vi "Main UI (ext control).vi"(0 "Serial port":refnum<visa-resource-name>="COM1", 1 "Command":T2, 5 "Data rate (Hz)":dbl=100.0, 7 "Max. num. sensors (override)":u8=64 max=64, 9 "Wait for HW trigger":bool, 11 "Finite samples":bool=TRUE, 12 "N samples":u32=1000, 14 "Error in":errorcluster) -> (4 "P data (mode 0)":T8[](array[typedef]), 15 "Error out":errorcluster)   [LabVIEW 2020]
doc: "User interface for 64 pressure multiplexer system designed by Paul Nathan, 02/2016"
uses:
  Ctls/System status.ctl
  Ctls/Environmental state values.ctl
  Ctls/Inertial state values.ctl
  Ctls/AccelGyro constants.ctl
  Ctls/Pressure sensor constants.ctl
  Ctls/Cmd list.ctl
  Ctls/Data values, Mode 0 (for datalog).ctl
  Ctls/All state values (for datalog).ctl
  Ctls/Cmd str.ctl
  Ctls/Data values, Mode 1 (for datalog).ctl
panel:
  in  "Main tabs":T1(tab)
  in  "Env. period (ms)":i32=1000 min=0
  out "ACK 8":bool caption="ACK"
  out "ACK 7":bool caption="ACK"
  out "ACK 6":bool caption="ACK"
  out "AccelGyro constants":T3={"gyrRange"=125.0, "accRange"=2.0, "gx offset"=0.0, "gy offset"=0.0, "gz offset"=0.0, "ax offset"=0.0, "ay offset"=0.0, "az offset"=0.0, "axyz scale"=1.0} {"axyz scale" format="%#_4f"; "az offset" format="%#_4f"; "ay offset" format="%#_4f"; "ax offset" format="%#_4f"; "gz offset" format="%#_4f"; "gy offset" format="%#_4f"; "gx offset" format="%#_4f"; "gyrRange" format="%#_4f"; "accRange" format="%#_4f"}
  out "Faulty sensors":i32[](array[numeric])
  out "ACK 5":bool caption="ACK"
  out "Active sensors":i32[](array[numeric])
  out "ACK 4":bool caption="ACK"
  in  "Gyro. rate (Hz)":u8(ring) items=["6.25", "12.5", "25", "50", "100", "200", "400", "800", "1600", "3200"]
  in  "Gyro. range (dps)":u8(ring) items=["+/- 125", "+/- 250", "+/- 500", "+/- 1000", "+/- 2000"]
  in  "Accel. rate (Hz)":u8(ring)=1 items=["3.125", "6.25", "12.5", "25", "50", "100", "200", "400", "800", "1600"]
  in  "Accel. range (g)":u8(ring) items=["+/- 2", "+/- 4", "+/- 8", "+/- 16"]
  out "Inertial state values":T4 {"w_z (dps)" format="%#_4f"; "a_y (g)" format="%#_4f"; "a_z (g)" format="%#_4f"; "w_y (dps)" format="%#_4f"; "a_x (g)" format="%#_4f"; "Sensor temp. (degC)" format="%#.2f"; "w_x (dps)" format="%#_4f"}
  out "Environmental state values":T5 {"Dew point (degC)" format="%#.2f"; "Density (kg/m^3)" format="%#.3f"; "Pressure alt. (m)" format="%#.2f"; "Density alt. (m)" format="%#.2f"; "Rel. Humidity (%)" format="%#.2f"; "P_atmos (Pa)" format="%#_6f"; "Sensor temp. (degC)" format="%#.2f"; "Thermistor (degC)" format="%#.2f"}
  out "System status":T6
  out "ACK 3":bool caption="ACK"
  out "ACK 1":bool caption="ACK"
  in  "Data mode":u8(ring) items=["P", "P & T"]
  out "ACK 2":bool caption="ACK"
  out "Main Power":bool
  out "L_data (bytes)":u16
  out "Serial no.":u16 format="%04x"
  out "Active pressure sensor constants":T7[](array[typedef])
  out "Streaming":bool
  out "Clock drift":bool
  out "Sensor temperatures time trace (Mode \"P & T\" only)":sgl[][](graph)
  out "Pressures time trace":sgl[][](graph)
  in  "Stop streaming":bool
  out "Stale samples flag":u8[][](graph)
  out "Samples acquired":u32
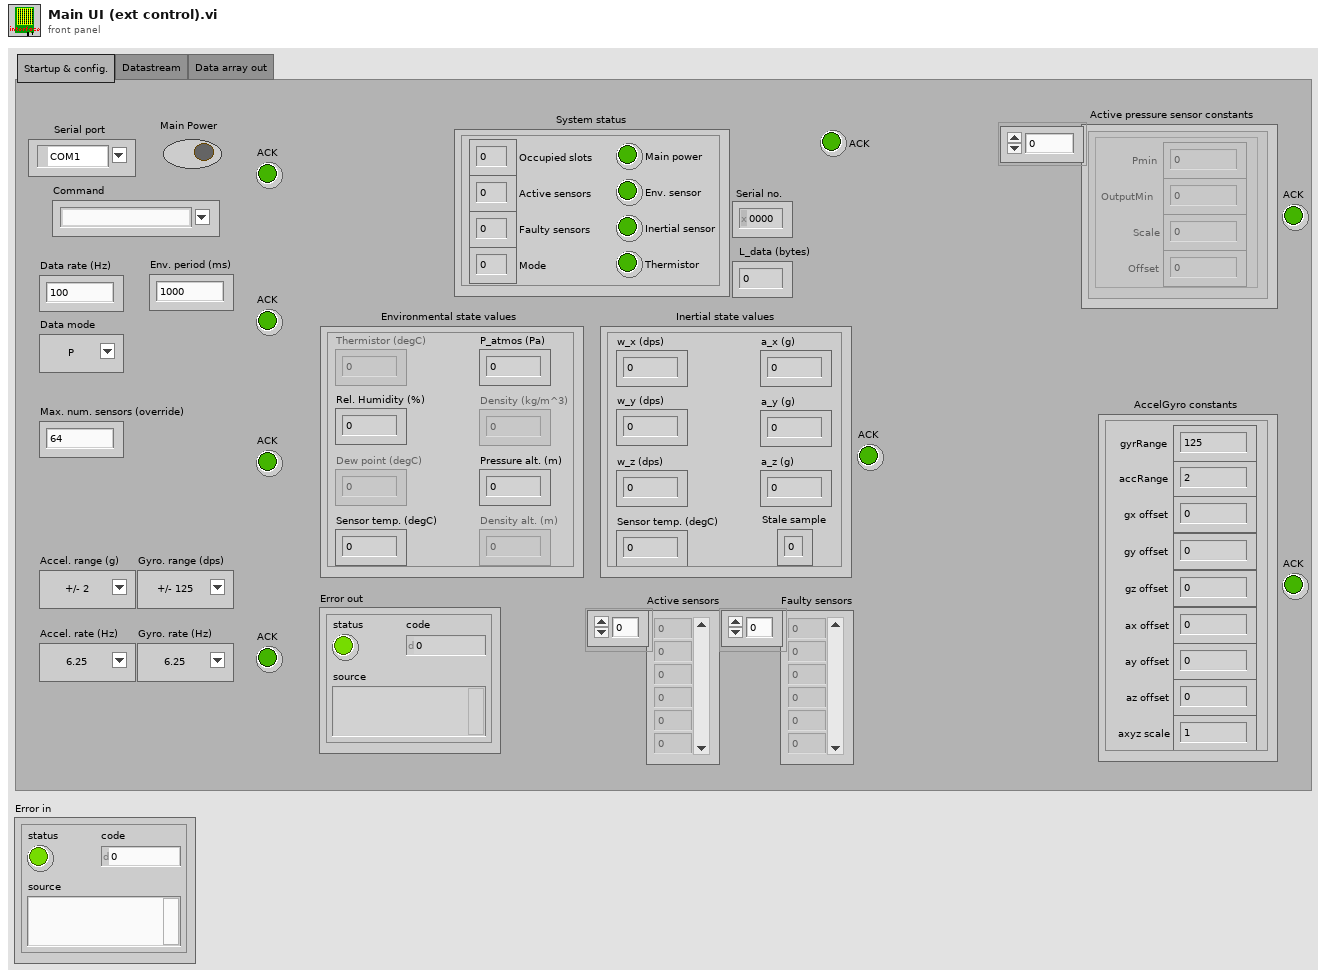
[diagram p1: front panel]
types:
  T1 = enum32{"Startup & config.", "Datastream", "Data array out"}
  T2 = typedef "Cmd list.ctl" = string
  T3 = typedef "AccelGyro constants.ctl" = cluster{"gyrRange":sgl, "accRange":sgl, "gx offset":sgl, "gy offset":sgl, "gz offset":sgl, "ax offset":sgl, "ay offset":sgl, "az offset":sgl, "axyz scale":sgl}
  T4 = typedef "Inertial state values.ctl" = cluster{"w_x (dps)":sgl, "w_y (dps)":sgl, "w_z (dps)":sgl, "a_x (g)":sgl, "a_y (g)":sgl, "a_z (g)":sgl, "Stale sample":u8, "Sensor temp. (degC)":sgl}
  T5 = typedef "Environmental state values.ctl" = cluster{"Thermistor (degC)":sgl, "Sensor temp. (degC)":sgl, "P_atmos (Pa)":sgl, "Rel. Humidity (%)":sgl, "Density (kg/m^3)":sgl, "Dew point (degC)":sgl, "Pressure alt. (m)":sgl, "Density alt. (m)":sgl}
  T6 = typedef "System status.ctl" = cluster{"Main power":bool, "Occupied slots":u8, "Active sensors":u8, "Faulty sensors":u8, "Env. sensor":bool, "Inertial sensor":bool, "Thermistor":bool, "Mode":u8}
  T7 = typedef "Pressure sensor constants.ctl" = cluster{"Pmin":sgl, "OutputMin":sgl, "Scale":sgl, "Offset":sgl}
  T8 = typedef "Data values, Mode 0 (for datalog).ctl" = cluster{"Time Stamp":timestamp, "dt (us)":sgl, "dt_warn":u8, "Pressures":sgl[], "Statuses":u8[]}
  T9 = typedef "All state values (for datalog).ctl" = cluster{"Time Stamp":timestamp, "dt (ms)":i32, "Environmental state values":T5, "Inertial state values":T4}
  T10 = typedef "Cmd str.ctl" = string
  T11 = typedef "Data values, Mode 1 (for datalog).ctl" = cluster{"Time Stamp":timestamp, "dt (us)":sgl, "dt_warn":u8, "Pressures":sgl[], "Die temps.":sgl[], "Statuses":u8[]}
  T12 = enum8{"Enabled", "Disabled", "Disabled and Grayed Out"}
  T13 = typedef "EEPROM page.ctl" = cluster{"Pmin (Pa)":sgl, "Pmax (Pa)":sgl, "maxCount":u16, "minCount":u16, "Poffset (Pa)":sgl}
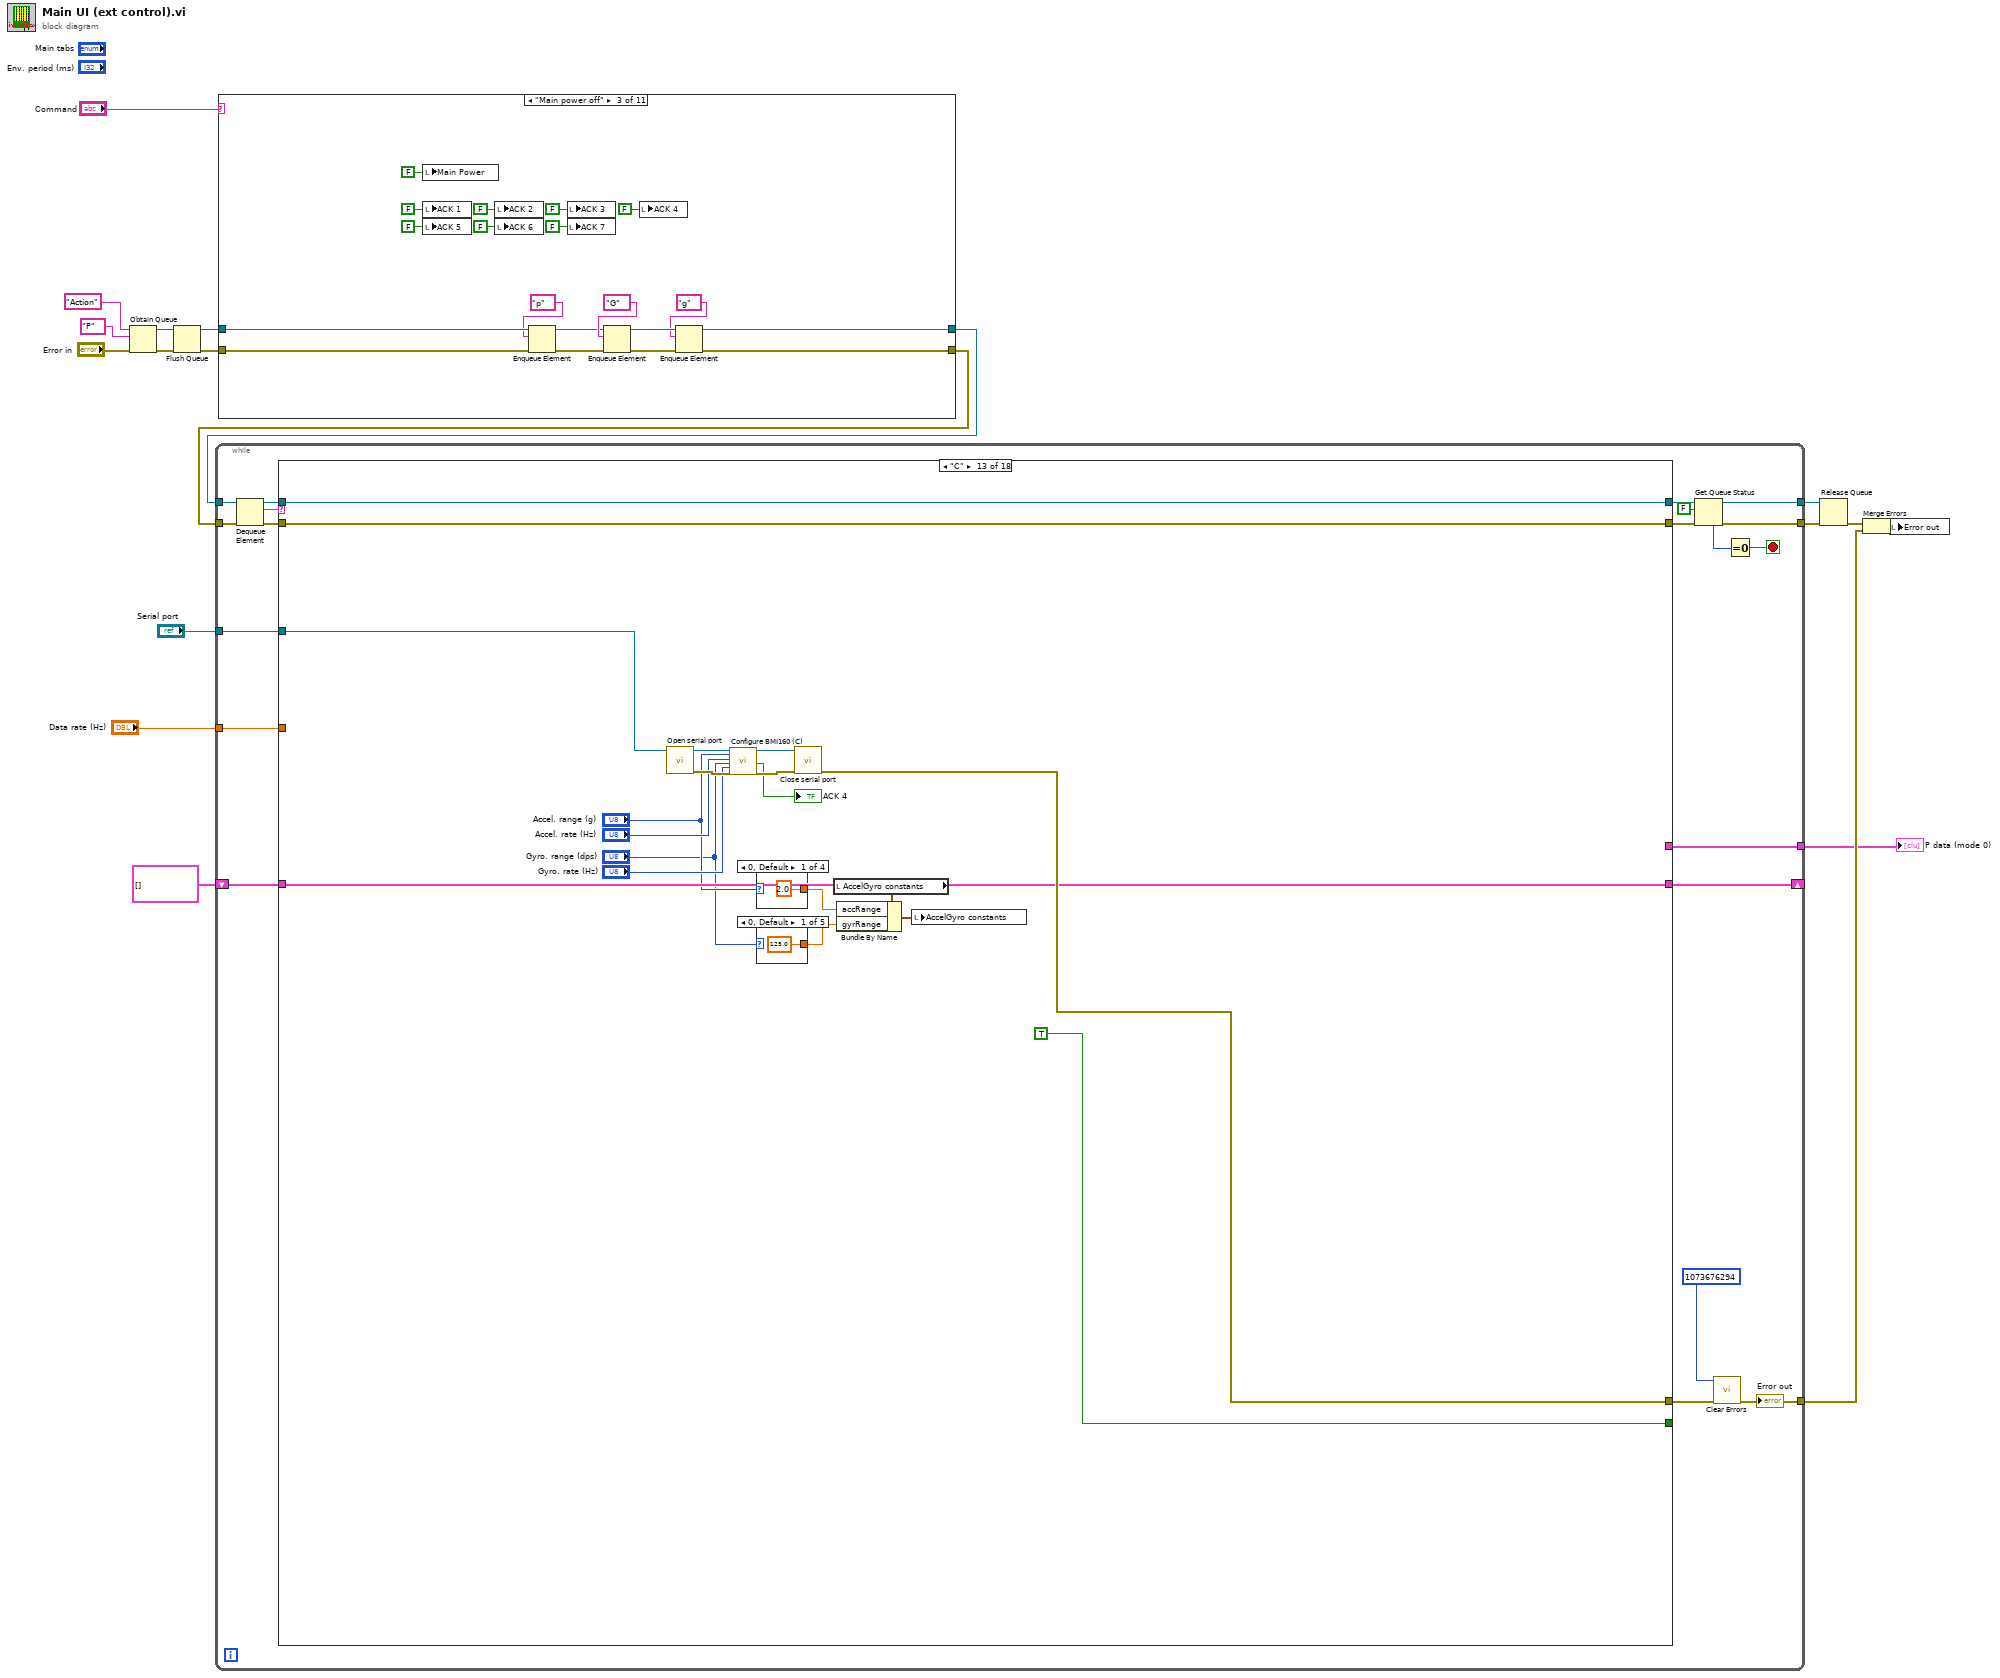
[diagram p0: block diagram]
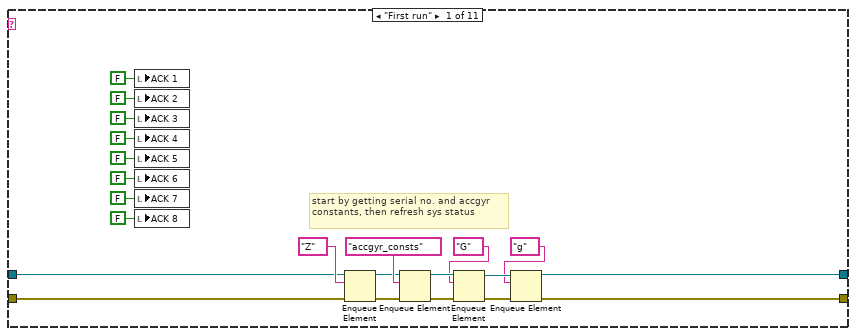
[diagram p2: hidden frame]
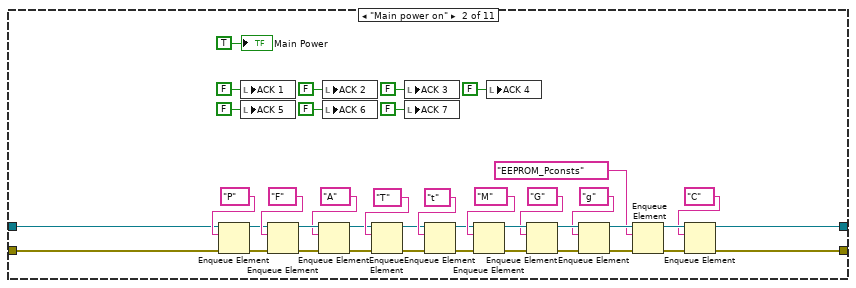
[diagram p3: hidden frame]
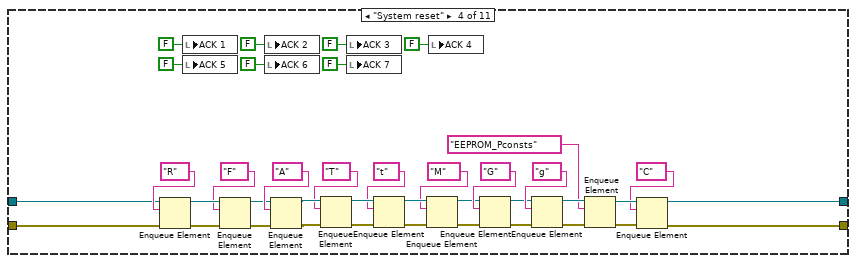
[diagram p4: hidden frame]
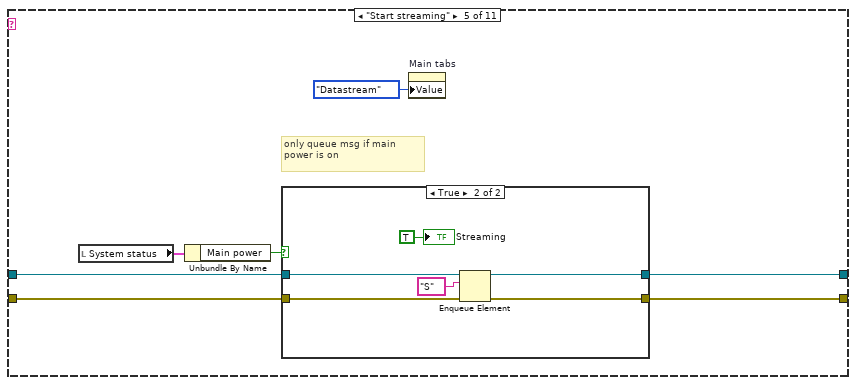
[diagram p5: hidden frame]
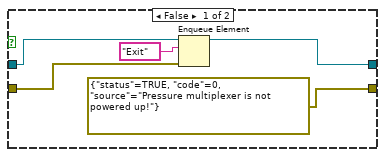
[diagram p6: hidden frame]
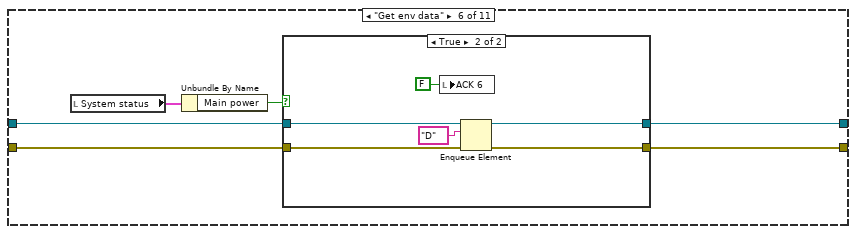
[diagram p7: hidden frame]
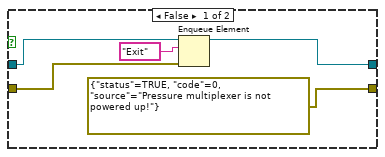
[diagram p8: hidden frame]
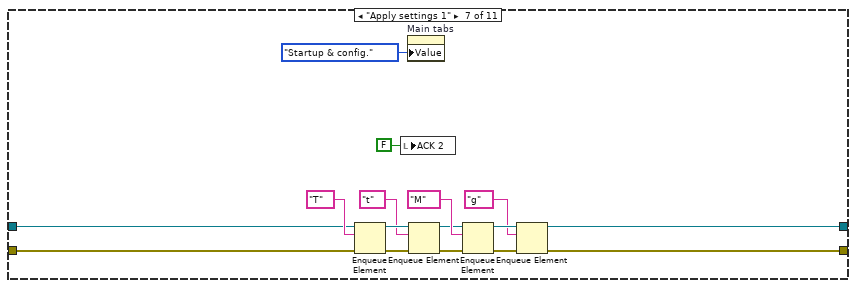
[diagram p9: hidden frame]
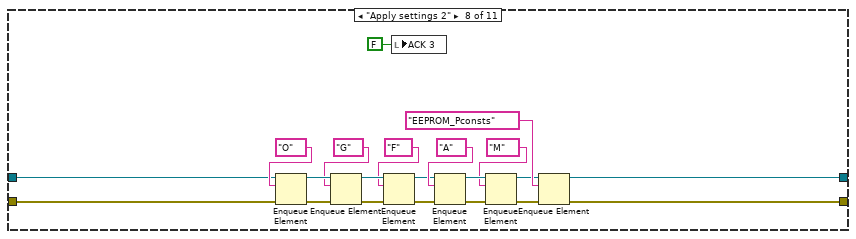
[diagram p10: hidden frame]
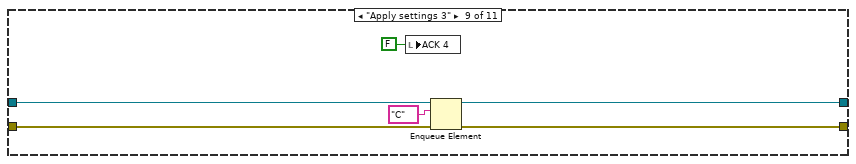
[diagram p11: hidden frame]
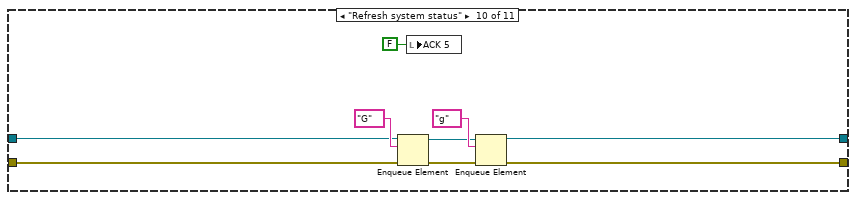
[diagram p12: hidden frame]
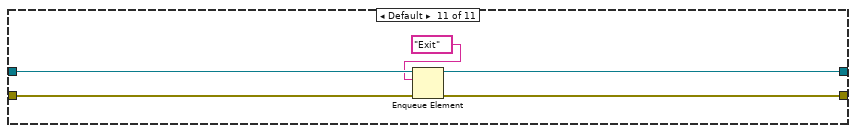
[diagram p13: hidden frame]
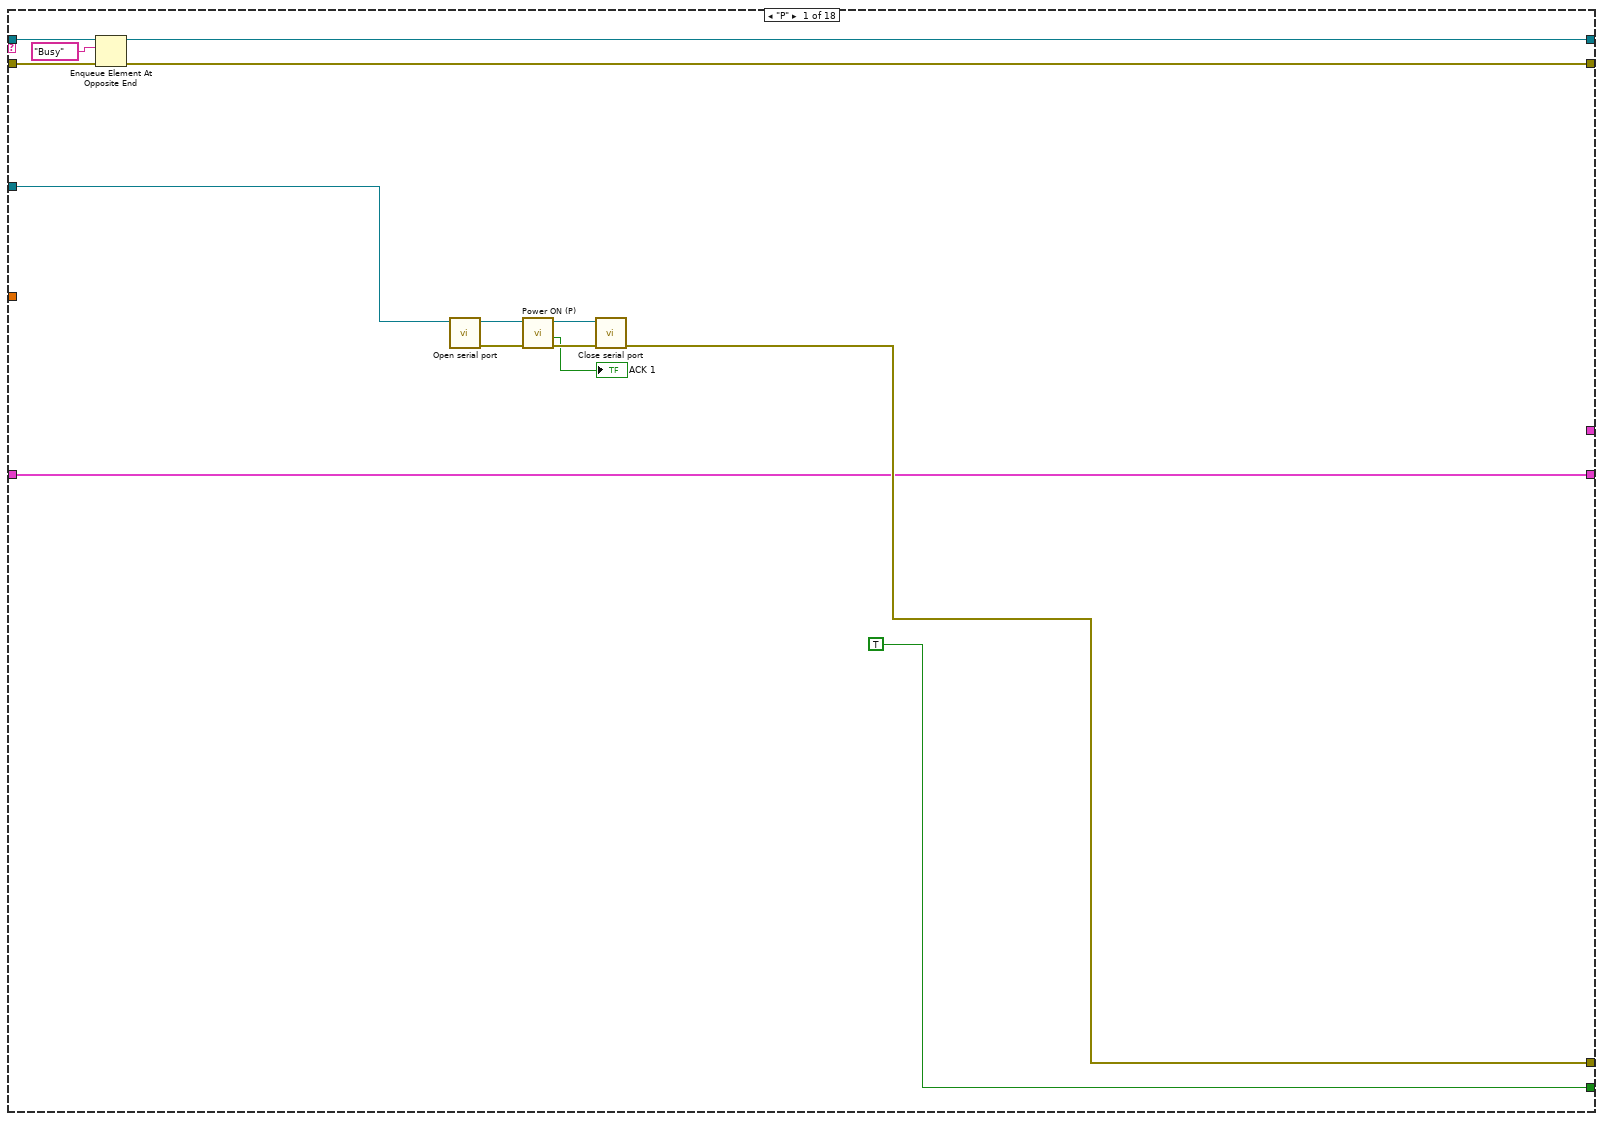
[diagram p14: hidden frame]
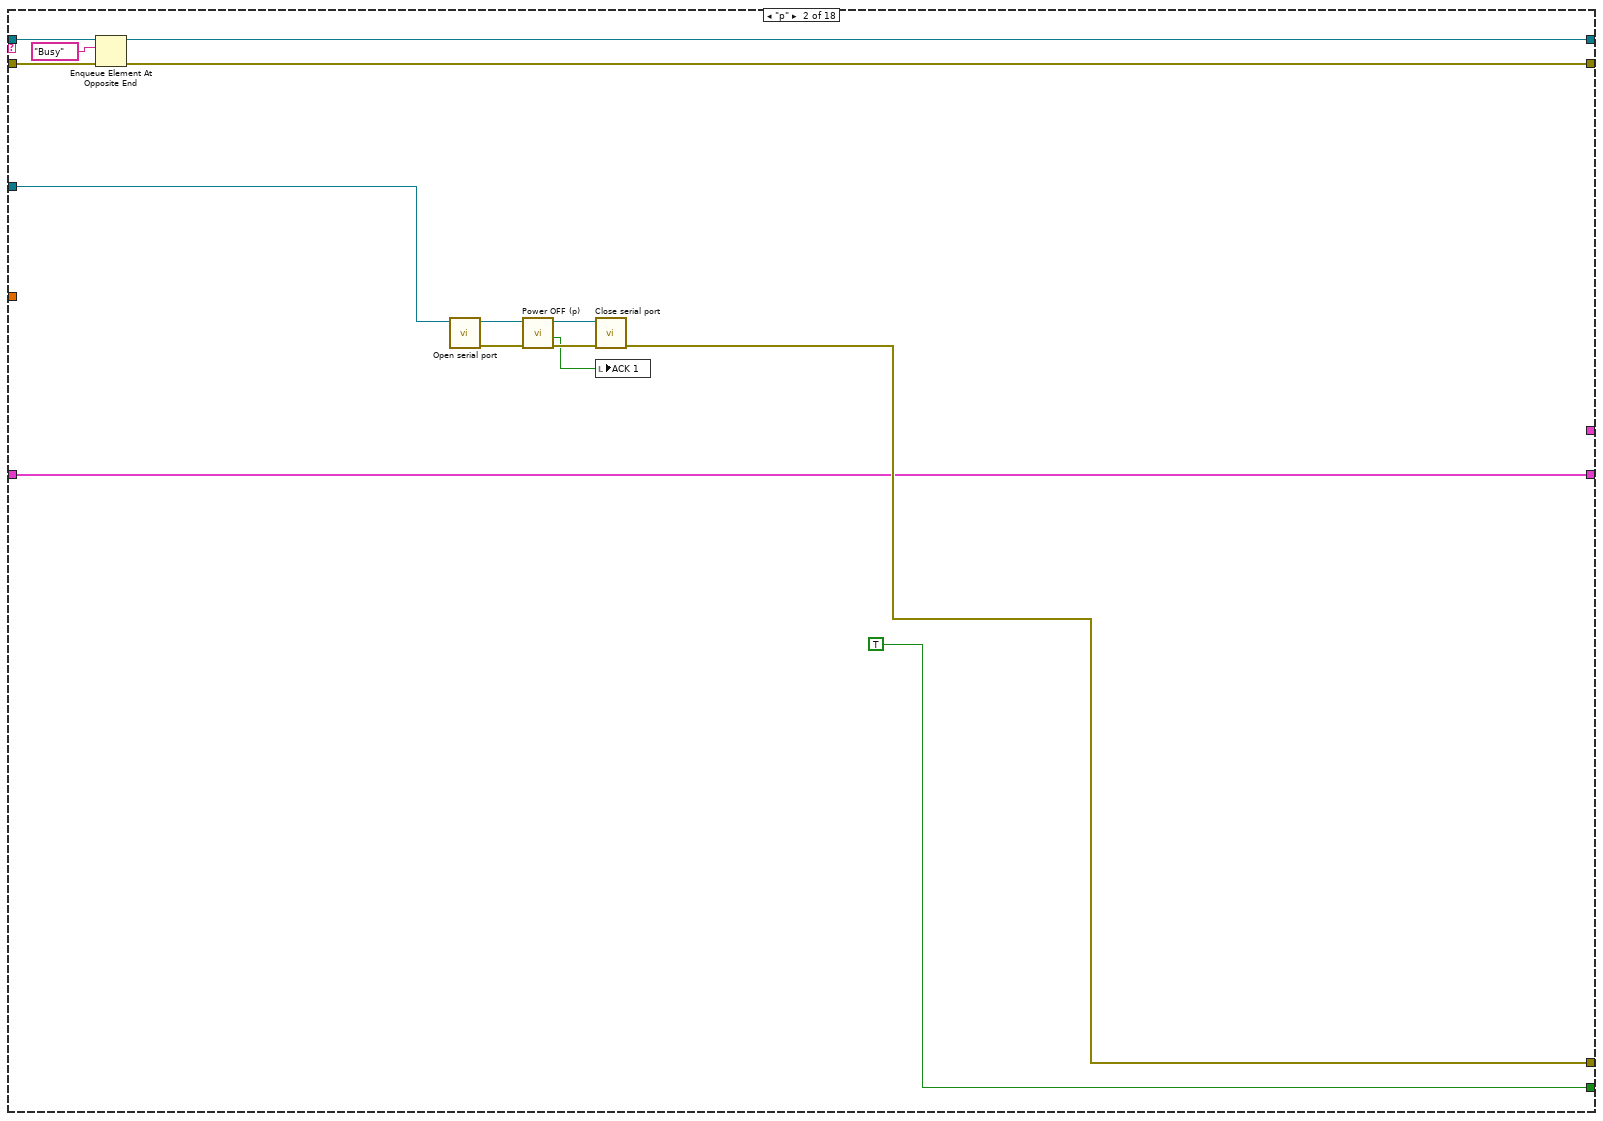
[diagram p15: hidden frame]
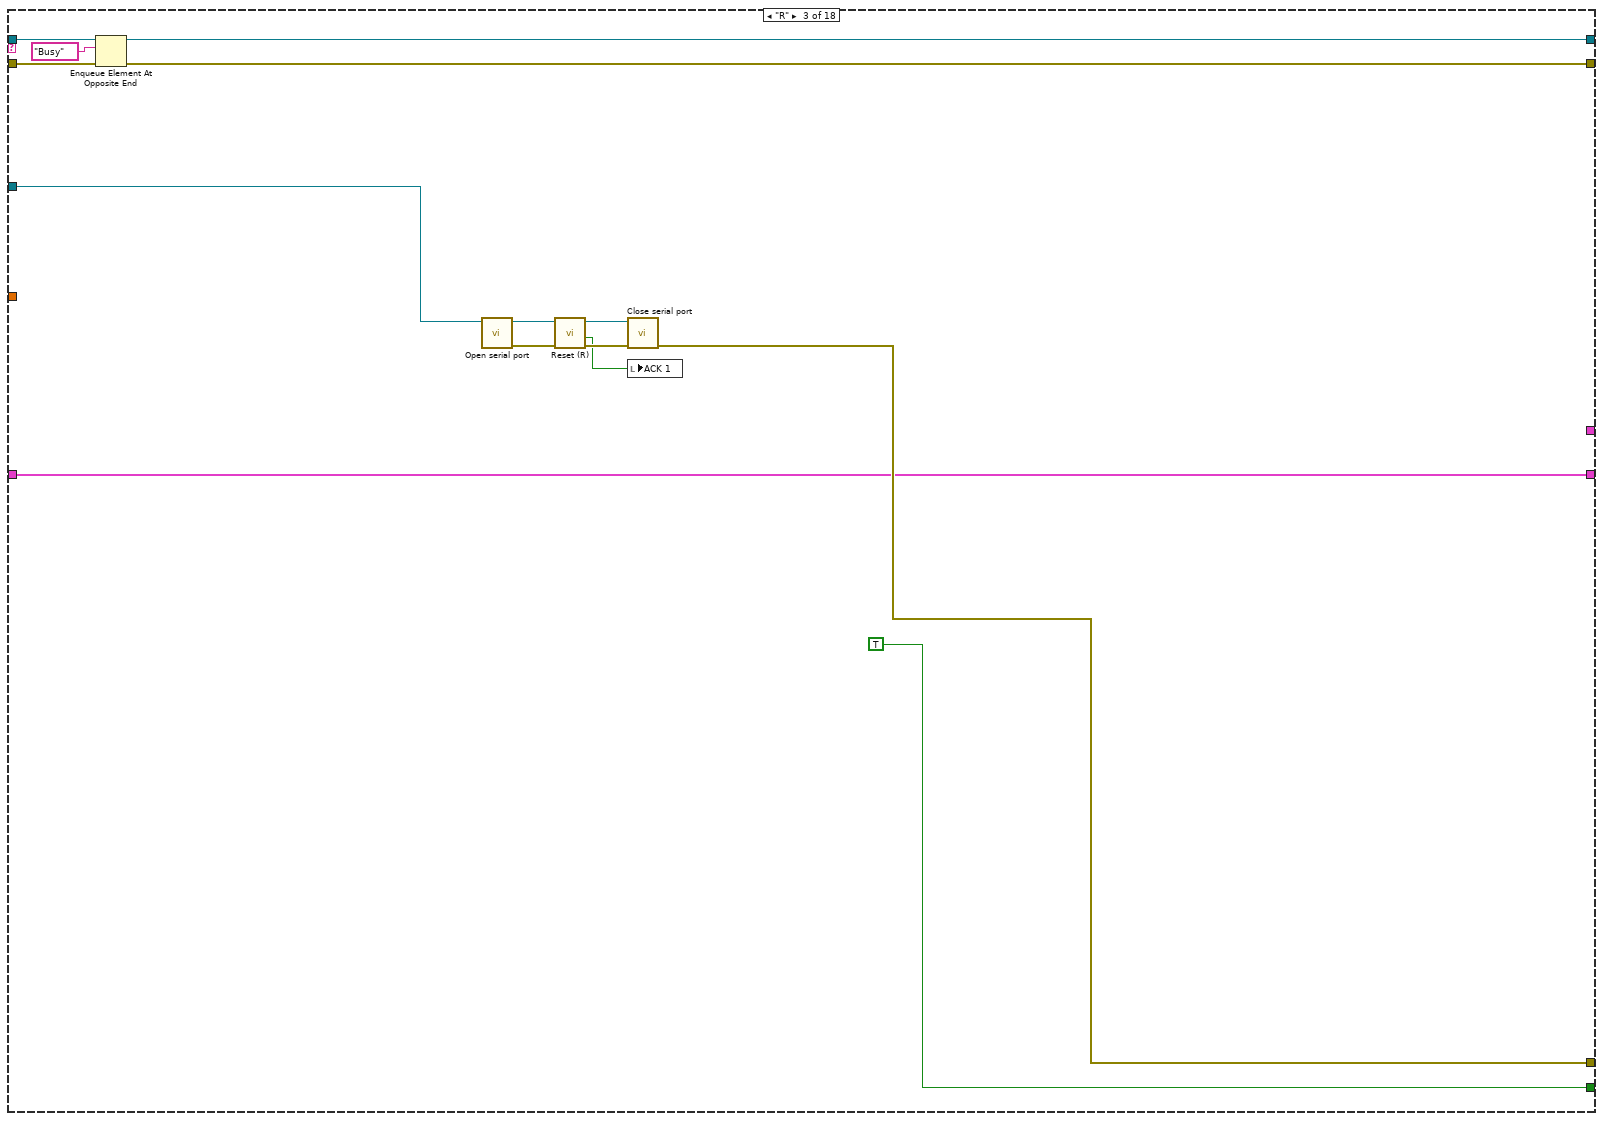
[diagram p16: hidden frame]
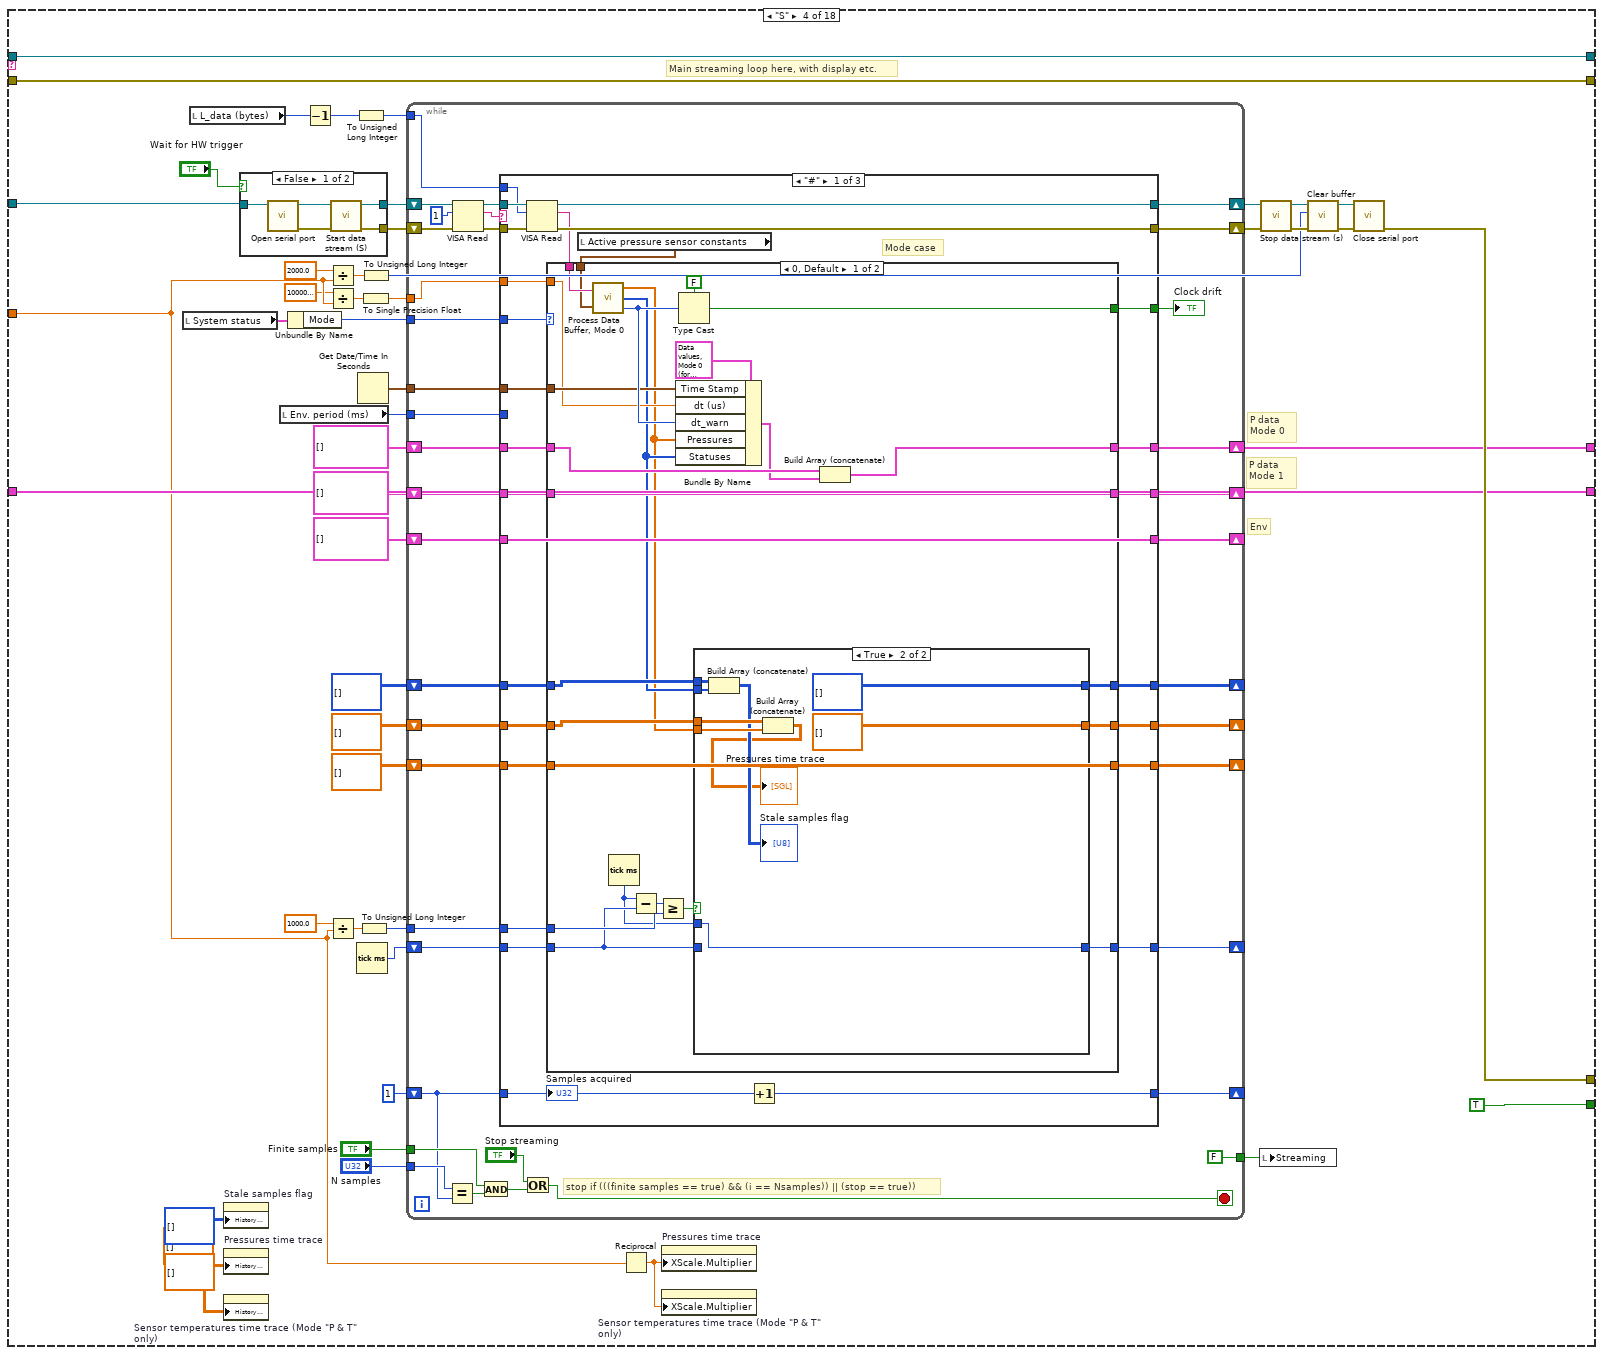
[diagram p17: hidden frame]
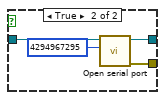
[diagram p18: hidden frame]
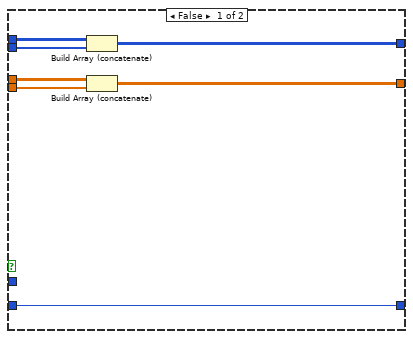
[diagram p19: hidden frame]
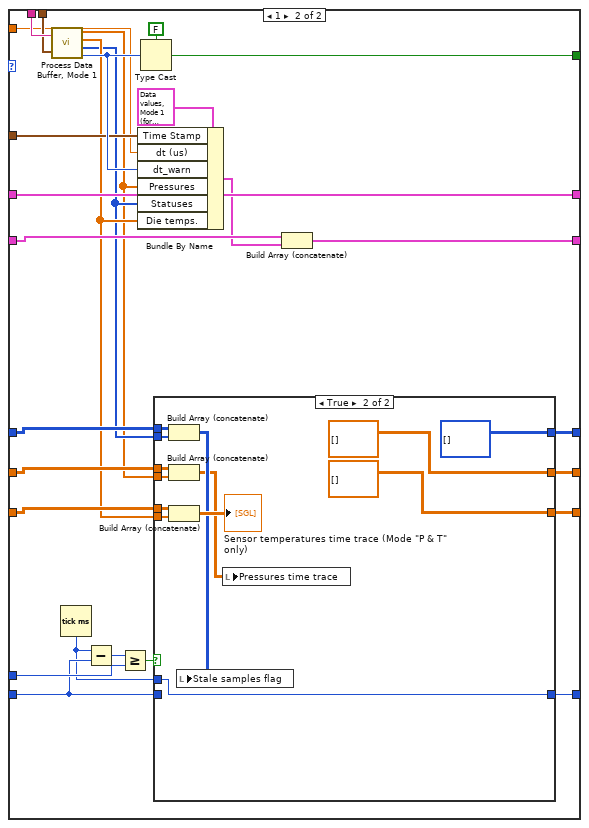
[diagram p20: hidden frame]
diagram:
  n1 = Obtain Queue(name (unnamed)="Action", element data type=T10 "P" ("Cmd"), error in (no error)="Error in") -> (queue out=w18:refnum<queue>, error out=w17:errorcluster)  [unwired: 2 in, 1 out]
  n2 = Flush Queue(queue=w18, error in (no error)=w17) -> (queue out=w6:refnum<queue>, error out=w5:errorcluster)  [unwired: 1 out]
  n3 = case shown="\"Main power off\"" "Command" {
    tunnel: [w29 w52 w92 w109 w141 w160 w178 w193 w214 w219 w227] -> w9
    tunnel: w5 -> [w30 w79 w99 w110 w144 w161 w179 w194 w215 w222 w231]
    tunnel: w6 -> [w31 w80 w100 w111 w143 w162 w180 w195 w216 w221 w230]
    tunnel: [w28 w51 w91 w108 w142 w159 w177 w192 w213 w220 w228] -> w8
    frame "First run" {
      # "start by getting serial no. and accgyr constants, then refresh sys status"
      n4 = local write "ACK 1"(FALSE ("ACK 8")) -> ()
      n5 = local write "ACK 2"(FALSE ("ACK 6")) -> ()
      n6 = local write "ACK 3"(FALSE ("ACK 8")) -> ()
      n7 = local write "ACK 4"(FALSE ("Done")) -> ()
      n8 = local write "ACK 5"(FALSE ("ACK 8")) -> ()
      n9 = local write "ACK 6"(FALSE ("ACK 6")) -> ()
      n10 = local write "ACK 7"(FALSE ("ACK 6")) -> ()
      n11 = local write "ACK 8"(FALSE ("ACK 8")) -> ()
      n12 = Enqueue Element(queue=w31, element=T10 "Z", error in (no error)=w30) -> (queue out=w33:refnum<queue>, error out=w34:errorcluster)  [unwired: 1 in, 1 out]
      n13 = Enqueue Element(queue=w33, element=T10 "accgyr_consts", error in (no error)=w34) -> (queue out=w40:refnum<queue>, error out=w41:errorcluster)  [unwired: 1 in, 1 out]
      n14 = Enqueue Element(queue=w40, element=T10 "G" ("Cmd"), error in (no error)=w41) -> (queue out=w38:refnum<queue>, error out=w37:errorcluster)  [unwired: 1 in, 1 out]
      n15 = Enqueue Element(queue=w38, element=T10 "g" ("Cmd"), error in (no error)=w37) -> (queue out=w28:refnum<queue>, error out=w29:errorcluster)  [unwired: 1 in, 1 out]
    }
    frame "Main power on" {
      n16 = Enqueue Element(queue=w80, element=T10 "P" ("Cmd"), error in (no error)=w79) -> (queue out=w73:refnum<queue>, error out=w72:errorcluster)  [unwired: 1 in, 1 out]
      n17 = local write "ACK 1"(FALSE ("ACK 1")) -> ()
      n18 = local write "ACK 5"(FALSE ("ACK 8")) -> ()
      n19 = Enqueue Element(queue=w73, element=T10 "F" ("Cmd"), error in (no error)=w72) -> (queue out=w77:refnum<queue>, error out=w78:errorcluster)  [unwired: 1 in, 1 out]
      n20 = Enqueue Element(queue=w77, element=T10 "A" ("Cmd"), error in (no error)=w78) -> (queue out=w58:refnum<queue>, error out=w57:errorcluster)  [unwired: 1 in, 1 out]
      n21 = local write "ACK 2"(FALSE ("ACK 6")) -> ()
      n22 = local write "ACK 6"(FALSE ("ACK 6")) -> ()
      n23 = Enqueue Element(queue=w58, element=T10 "T" ("Cmd"), error in (no error)=w57) -> (queue out=w60:refnum<queue>, error out=w59:errorcluster)  [unwired: 1 in, 1 out]
      n24 = local write "ACK 3"(FALSE ("ACK 8")) -> ()
      n25 = local write "ACK 7"(FALSE ("ACK 6")) -> ()
      n26 = Enqueue Element(queue=w60, element=T10 "t" ("Cmd"), error in (no error)=w59) -> (queue out=w55:refnum<queue>, error out=w56:errorcluster)  [unwired: 1 in, 1 out]
      n27 = Enqueue Element(queue=w55, element=T10 "M" ("Cmd"), error in (no error)=w56) -> (queue out=w69:refnum<queue>, error out=w68:errorcluster)  [unwired: 1 in, 1 out]
      n28 = local write "ACK 4"(FALSE ("Done")) -> ()
      n29 = Enqueue Element(queue=w69, element=T10 "G" ("Cmd"), error in (no error)=w68) -> (queue out=w70:refnum<queue>, error out=w71:errorcluster)  [unwired: 1 in, 1 out]
      n30 = Enqueue Element(queue=w70, element=T10 "g" ("Cmd"), error in (no error)=w71) -> (queue out=w65:refnum<queue>, error out=w64:errorcluster)  [unwired: 1 in, 1 out]
      n31 = Enqueue Element(queue=w65, element=T10 "EEPROM_Pconsts" ("Cmd"), error in (no error)=w64) -> (queue out=w54:refnum<queue>, error out=w53:errorcluster)  [unwired: 1 in, 1 out]
      n32 = Enqueue Element(queue=w54, element=T10 "C" ("Cmd"), error in (no error)=w53) -> (queue out=w51:refnum<queue>, error out=w52:errorcluster)  [unwired: 1 in, 1 out]
      "Main Power" <- TRUE ("Main Power")
    }
    frame "Main power off" {
      n33 = local write "Main Power"(FALSE ("Main Power")) -> ()
      n34 = local write "ACK 1"(FALSE ("ACK 1")) -> ()
      n35 = local write "ACK 5"(FALSE ("ACK 8")) -> ()
      n36 = local write "ACK 2"(FALSE ("ACK 6")) -> ()
      n37 = local write "ACK 6"(FALSE ("ACK 6")) -> ()
      n38 = Enqueue Element(queue=w100, element=T10 "p" ("Cmd"), error in (no error)=w99) -> (queue out=w96:refnum<queue>, error out=w95:errorcluster)  [unwired: 1 in, 1 out]
      n39 = local write "ACK 3"(FALSE ("ACK 8")) -> ()
      n40 = local write "ACK 7"(FALSE ("ACK 6")) -> ()
      n41 = Enqueue Element(queue=w96, element=T10 "G" ("Cmd"), error in (no error)=w95) -> (queue out=w94:refnum<queue>, error out=w93:errorcluster)  [unwired: 1 in, 1 out]
      n42 = local write "ACK 4"(FALSE ("Done")) -> ()
      n43 = Enqueue Element(queue=w94, element=T10 "g" ("Cmd"), error in (no error)=w93) -> (queue out=w91:refnum<queue>, error out=w92:errorcluster)  [unwired: 1 in, 1 out]
    }
    frame "System reset" {
      n44 = Enqueue Element(queue=w111, element=T10 "R" ("Cmd"), error in (no error)=w110) -> (queue out=w123:refnum<queue>, error out=w124:errorcluster)  [unwired: 1 in, 1 out]
      n45 = local write "ACK 1"(FALSE ("ACK 1")) -> ()
      n46 = local write "ACK 5"(FALSE ("ACK 8")) -> ()
      n47 = Enqueue Element(queue=w123, element=T10 "F" ("Cmd"), error in (no error)=w124) -> (queue out=w115:refnum<queue>, error out=w125:errorcluster)  [unwired: 1 in, 1 out]
      n48 = local write "ACK 2"(FALSE ("ACK 6")) -> ()
      n49 = local write "ACK 6"(FALSE ("ACK 6")) -> ()
      n50 = Enqueue Element(queue=w115, element=T10 "A" ("Cmd"), error in (no error)=w125) -> (queue out=w133:refnum<queue>, error out=w134:errorcluster)  [unwired: 1 in, 1 out]
      n51 = Enqueue Element(queue=w133, element=T10 "T" ("Cmd"), error in (no error)=w134) -> (queue out=w131:refnum<queue>, error out=w132:errorcluster)  [unwired: 1 in, 1 out]
      n52 = local write "ACK 3"(FALSE ("ACK 8")) -> ()
      n53 = local write "ACK 7"(FALSE ("ACK 6")) -> ()
      n54 = Enqueue Element(queue=w131, element=T10 "t" ("Cmd"), error in (no error)=w132) -> (queue out=w135:refnum<queue>, error out=w136:errorcluster)  [unwired: 1 in, 1 out]
      n55 = Enqueue Element(queue=w135, element=T10 "M" ("Cmd"), error in (no error)=w136) -> (queue out=w119:refnum<queue>, error out=w126:errorcluster)  [unwired: 1 in, 1 out]
      n56 = local write "ACK 4"(FALSE ("Done")) -> ()
      n57 = Enqueue Element(queue=w119, element=T10 "G" ("Cmd"), error in (no error)=w126) -> (queue out=w118:refnum<queue>, error out=w127:errorcluster)  [unwired: 1 in, 1 out]
      n58 = Enqueue Element(queue=w118, element=T10 "g" ("Cmd"), error in (no error)=w127) -> (queue out=w122:refnum<queue>, error out=w128:errorcluster)  [unwired: 1 in, 1 out]
      n59 = Enqueue Element(queue=w122, element=T10 "EEPROM_Pconsts" ("Cmd"), error in (no error)=w128) -> (queue out=w138:refnum<queue>, error out=w139:errorcluster)  [unwired: 1 in, 1 out]
      n60 = Enqueue Element(queue=w138, element=T10 "C" ("Cmd"), error in (no error)=w139) -> (queue out=w108:refnum<queue>, error out=w109:errorcluster)  [unwired: 1 in, 1 out]
    }
    frame "Start streaming" {
      # "only queue msg if main power is on"
      n61 = local read "System status"() -> (w146:T6)
      n62 = Unbundle By Name(w146) -> ("Main power"=w145:bool)
      n63 = case shown="True" w145 {
        tunnel: w143 -> [w149 w156]
        tunnel: w144 -> [w147 w155]
        tunnel: [w148 w153] -> w142
        tunnel: [errorcluster {"status"=TRUE, "code"=0, "source"="Pressure multiplexer is not powered up!"} ("error out") w154] -> w141
        frame False {
          n64 = Enqueue Element(queue=w149, element=T10 "Exit" ("Cmd"), error in (no error)=w147) -> (queue out=w148:refnum<queue>)  [unwired: 1 in, 2 out]
        }
        frame True {
          n65 = Enqueue Element(queue=w156, element=T10 "S" ("Cmd"), error in (no error)=w155) -> (queue out=w153:refnum<queue>, error out=w154:errorcluster)  [unwired: 1 in, 1 out]
          "Streaming" <- TRUE ("Streaming")
        }
      }
      n66 = property on="Main tabs" class="TabCtl (strict)"("Value"=T1."Datastream" ("Main tabs")) -> ()  [unwired: 2 in, 2 out]
    }
    frame "Get env data" {
      n67 = local read "System status"() -> (w163:T6)
      n68 = Unbundle By Name(w163) -> ("Main power"=w158:bool)
      n69 = case shown="True" w158 {
        tunnel: w162 -> [w166 w173]
        tunnel: w161 -> [w164 w172]
        tunnel: [w165 w170] -> w159
        tunnel: [errorcluster {"status"=TRUE, "code"=0, "source"="Pressure multiplexer is not powered up!"} ("error out") w171] -> w160
        frame False {
          n70 = Enqueue Element(queue=w166, element=T10 "Exit" ("Cmd"), error in (no error)=w164) -> (queue out=w165:refnum<queue>)  [unwired: 1 in, 2 out]
        }
        frame True {
          n71 = local write "ACK 6"(FALSE ("ACK 6")) -> ()
          n72 = Enqueue Element(queue=w173, element=T10 "D" ("Cmd"), error in (no error)=w172) -> (queue out=w170:refnum<queue>, error out=w171:errorcluster)  [unwired: 1 in, 1 out]
        }
      }
    }
    frame "Apply settings 1" {
      n73 = Enqueue Element(queue=w180, element=T10 "T" ("Cmd"), error in (no error)=w179) -> (queue out=w183:refnum<queue>, error out=w184:errorcluster)  [unwired: 1 in, 1 out]
      n74 = local write "ACK 2"(FALSE ("ACK 6")) -> ()
      n75 = property on="Main tabs" class="TabCtl (strict)"("Value"=T1."Startup & config." ("Main tabs")) -> ()  [unwired: 2 in, 2 out]
      n76 = Enqueue Element(queue=w183, element=T10 "t" ("Cmd"), error in (no error)=w184) -> (queue out=w186:refnum<queue>, error out=w185:errorcluster)  [unwired: 1 in, 1 out]
      n77 = Enqueue Element(queue=w186, element=T10 "M" ("Cmd"), error in (no error)=w185) -> (queue out=w189:refnum<queue>, error out=w190:errorcluster)  [unwired: 1 in, 1 out]
      n78 = Enqueue Element(queue=w189, element=T10 "g" ("Cmd"), error in (no error)=w190) -> (queue out=w177:refnum<queue>, error out=w178:errorcluster)  [unwired: 1 in, 1 out]
    }
    frame "Apply settings 2" {
      n79 = Enqueue Element(queue=w195, element=T10 "O" ("Cmd"), error in (no error)=w194) -> (queue out=w198:refnum<queue>, error out=w199:errorcluster)  [unwired: 1 in, 1 out]
      n80 = Enqueue Element(queue=w198, element=T10 "G" ("Cmd"), error in (no error)=w199) -> (queue out=w210:refnum<queue>, error out=w211:errorcluster)  [unwired: 1 in, 1 out]
      n81 = Enqueue Element(queue=w210, element=T10 "F" ("Cmd"), error in (no error)=w211) -> (queue out=w206:refnum<queue>, error out=w205:errorcluster)  [unwired: 1 in, 1 out]
      n82 = local write "ACK 3"(FALSE ("ACK 8")) -> ()
      n83 = Enqueue Element(queue=w206, element=T10 "A" ("Cmd"), error in (no error)=w205) -> (queue out=w208:refnum<queue>, error out=w209:errorcluster)  [unwired: 1 in, 1 out]
      n84 = Enqueue Element(queue=w208, element=T10 "M" ("Cmd"), error in (no error)=w209) -> (queue out=w201:refnum<queue>, error out=w200:errorcluster)  [unwired: 1 in, 1 out]
      n85 = Enqueue Element(queue=w201, element=T10 "EEPROM_Pconsts" ("Cmd"), error in (no error)=w200) -> (queue out=w192:refnum<queue>, error out=w193:errorcluster)  [unwired: 1 in, 1 out]
    }
    frame "Apply settings 3" {
      n86 = local write "ACK 4"(FALSE ("Done")) -> ()
      n87 = Enqueue Element(queue=w216, element=T10 "C" ("Cmd"), error in (no error)=w215) -> (queue out=w213:refnum<queue>, error out=w214:errorcluster)  [unwired: 1 in, 1 out]
    }
    frame "Refresh system status" {
      n88 = Enqueue Element(queue=w221, element=T10 "G" ("Cmd"), error in (no error)=w222) -> (queue out=w224:refnum<queue>, error out=w225:errorcluster)  [unwired: 1 in, 1 out]
      n89 = local write "ACK 5"(FALSE ("ACK 8")) -> ()
      n90 = Enqueue Element(queue=w224, element=T10 "g" ("Cmd"), error in (no error)=w225) -> (queue out=w220:refnum<queue>, error out=w219:errorcluster)  [unwired: 1 in, 1 out]
    }
    frame Default {
      n91 = Enqueue Element(queue=w230, element=T10 "Exit" ("Cmd"), error in (no error)=w231) -> (queue out=w228:refnum<queue>, error out=w227:errorcluster)  [unwired: 1 in, 1 out]
    }
  }
  n92 = while {
    tunnel: w9 -> [w250]
    tunnel: w8 -> [w251]
    tunnel: [w238] -> w16
    shift-right: [w246] -> _
    shift-left: T9[] [] -> [w245]
    tunnel: [w242] -> w12
    tunnel: [w235] -> w10
    tunnel: [w234] -> w4
    tunnel: "Serial port" -> [w233]
    tunnel: "Data rate (Hz)" -> [w232]
    stop <- w236 stop-if-true
    n93 = Dequeue Element(queue=w251, error in (no error)=w250) -> (queue out=w249:refnum<queue>, element=w247:T10, error out=w248:errorcluster)  [unwired: 1 in, 1 out]
    n94 = case shown="\"C\"" w247 {
      tunnel: w249 -> [w265 w279 w293 w338 w554 w567 w580 w593 w610 w632 w647 w658 w677 w697 w719 w740 w757 w758]
      tunnel: w248 -> [w264 w278 w292 w337 w553 w566 w579 w592 w609 w631 w646 w657 w676 w696 w718 w739 w756 w762]
      tunnel: [w262 w276 w290 w337 w553 w566 w579 w592 w609 w631 w646 w657 w676 w696 w718 w739 w756 w762] -> w240
      tunnel: [TRUE TRUE TRUE TRUE TRUE TRUE TRUE TRUE TRUE TRUE TRUE TRUE TRUE TRUE TRUE TRUE TRUE FALSE] -> _
      tunnel: [w260 w274 w288 w340 w551 w564 w577 w590 w607 w629 w644 w655 w674 w694 w716 w737 w754 errorcluster {"status"=FALSE, "code"=0, "source"=""} ("Error out")] -> w243
      tunnel: [w258 w272 w286 w339 w550 w563 w576 w589 w606 w628 w643 w654 w673 w693 w715 w736 w753 w759] -> w246
      tunnel: w245 -> [w258 w272 w286 w339 w550 w563 w576 w589 w606 w628 w643 w654 w673 w693 w714 w736 w753 w759]
      tunnel: [w263 w277 w291 w338 w554 w567 w580 w593 w610 w632 w647 w658 w677 w697 w719 w740 w757 w758] -> w241
      tunnel: [_ _ _ w336 _ _ _ _ _ _ _ _ _ _ _ _ _ _] -> w234
      tunnel: w233 -> [w257 w271 w285 w335 w548 w562 w568 w581 w594 w611 w637 w648 w659 w687 w698 w720 w741 _]
      tunnel: w232 -> [_ _ _ w334 w549 _ _ _ _ _ _ _ _ _ _ _ _ _]
      frame "P" {
        n95 = Enqueue Element At Opposite End(queue=w265, element=T10 "Busy" ("Cmd"), error in (no error)=w264) -> (queue out=w263:refnum<queue>, error out=w262:errorcluster)  [unwired: 1 in, 1 out]
        n96 = call "Open serial port.vi"("VISA resource name"=w257) -> ("Error out"=w255:errorcluster, "VISA resource name out"=w256:refnum<visa-resource-name>)  [unwired: 9 in]
        n97 = call "Power ON (P).vi"("Error In"=w255, "VISA resource name in"=w256) -> ("Error out"=w254:errorcluster, "ACK"=→"ACK 1":bool, "VISA resource name out"=w253:refnum<visa-resource-name>)  [unwired: 7 in]
        n98 = call "Close serial port.vi"("Error in"=w254, "VISA resource name"=w253) -> ("Error out"=w260:errorcluster)  [unwired: 9 in]
      }
      frame "p" {
        n99 = Enqueue Element At Opposite End(queue=w279, element=T10 "Busy" ("Cmd"), error in (no error)=w278) -> (queue out=w277:refnum<queue>, error out=w276:errorcluster)  [unwired: 1 in, 1 out]
        n100 = call "Open serial port.vi"("VISA resource name"=w271) -> ("Error out"=w269:errorcluster, "VISA resource name out"=w270:refnum<visa-resource-name>)  [unwired: 9 in]
        n101 = call "Power OFF (p).vi"("Error In"=w269, "VISA resource name in"=w270) -> ("Error out"=w268:errorcluster, "ACK"=w266:bool, "VISA resource name out"=w267:refnum<visa-resource-name>)  [unwired: 7 in]
        n102 = call "Close serial port.vi"("Error in"=w268, "VISA resource name"=w267) -> ("Error out"=w274:errorcluster)  [unwired: 9 in]
        n103 = local write "ACK 1"(w266) -> ()
      }
      frame "R" {
        n104 = Enqueue Element At Opposite End(queue=w293, element=T10 "Busy" ("Cmd"), error in (no error)=w292) -> (queue out=w291:refnum<queue>, error out=w290:errorcluster)  [unwired: 1 in, 1 out]
        n105 = call "Open serial port.vi"("VISA resource name"=w285) -> ("Error out"=w280:errorcluster, "VISA resource name out"=w281:refnum<visa-resource-name>)  [unwired: 9 in]
        n106 = call "Reset (R).vi"("Error In"=w280, "VISA resource name in"=w281) -> ("Error out"=w284:errorcluster, "ACK"=w282:bool, "VISA resource name out"=w283:refnum<visa-resource-name>)  [unwired: 7 in]
        n107 = call "Close serial port.vi"("Error in"=w284, "VISA resource name"=w283) -> ("Error out"=w288:errorcluster)  [unwired: 9 in]
        n108 = local write "ACK 1"(w282) -> ()
      }
      frame "S" {
        # "Env"
        # "P data Mode 1"
        # "P data Mode 0"
        # "Main streaming loop here, with display etc."
        n109 = local read "System status"() -> (w310:T6)
        n110 = local read "L_data (bytes)"() -> (w316:u16)
        n111 = property on="Stale samples flag" class="WFChart (strict)"("History Data"=u8[][] []) -> ()  [unwired: 2 in, 2 out]
        n112 = property on="Pressures time trace" class="WFChart (strict)"("History Data"=sgl[][] []) -> ()  [unwired: 2 in, 2 out]
        n113 = property on="Sensor temperatures time trace (Mode \"P & T\" only)" class="WFChart (strict)"("History Data"=sgl[][] []) -> ()  [unwired: 2 in, 2 out]
        n114 = case shown="False" "Wait for HW trigger" {
          tunnel: [w344 w348] -> w333
          tunnel: [w343 w349] -> w332
          tunnel: w335 -> [w342 w350]
          frame False {
            n115 = call "Open serial port.vi"("VISA resource name"=w342) -> ("Error out"=w345:errorcluster, "VISA resource name out"=w346:refnum<visa-resource-name>)  [unwired: 9 in]
            n116 = call "Start data stream (S).vi"("VISA resource name in"=w346, "Error In"=w345) -> ("VISA resource name out"=w343:refnum<visa-resource-name>, "Error out"=w344:errorcluster)  [unwired: 7 in]
          }
          frame True {
            n117 = call "Open serial port.vi"("timeout (ms)"=u32 4294967295, "VISA resource name"=w350) -> ("Error out"=w348:errorcluster, "VISA resource name out"=w349:refnum<visa-resource-name>)  [unwired: 8 in]
          }
        }
        n118 = local read "Env. period (ms)"() -> (w314:i32)
        n119 = Unbundle By Name(w310) -> ("Mode"=w300:u8)
        n120 = Decrement(x=w316) -> (x-1=w301:u16)
        n121 = Divide(x=2000.0 ("y"), y=w334) -> (x/y=w326:dbl)
        n122 = Divide(x=1000000.0 ("y"), y=w334) -> (x/y=w312:dbl)
        n123 = Divide(x=1000.0, y=w334) -> (x/y=w321:dbl)
        n124 = To Unsigned Long Integer(number=w301) -> (unsigned 32bit integer=w315:u32)
        n125 = Tick Count (ms)() -> (millisecond timer value=w302:u32)
        n126 = Get Date/Time In Seconds() -> (seconds since 1Jan1904=w331:timestamp)
        n127 = To Unsigned Long Integer(number=w321) -> (unsigned 32bit integer=w319:u32)
        n128 = To Unsigned Long Integer(number=w326) -> (unsigned 32bit integer=w325:u32)
        n129 = To Single Precision Float(number=w312) -> (single precision float=w311:sgl)
        n130 = while {
          shift-right: [w382] -> w329
          shift-left: w332 -> [w387]
          shift-right: [w381] -> w330
          shift-left: w333 -> [w388]
          tunnel: w331 -> [w380]
          tunnel: "Finite samples" -> [w377]
          tunnel: "N samples" -> [w379]
          shift-right: [w373] -> _
          shift-left: T9[] [] -> [w372]
          tunnel: w319 -> [w361]
          shift-right: [w368] -> _
          shift-left: T11[] [] -> [w370]
          shift-right: [w369] -> w336
          shift-left: T8[] [] -> [w371]
          tunnel: w315 -> [w367]
          tunnel: w314 -> [w366]
          tunnel: w311 -> [w365]
          tunnel: w300 -> [w354]
          shift-right: [w363] -> _
          shift-left: w302 -> [w362]
          shift-right: [w360] -> _
          shift-left: sgl[][] [] -> [w357]
          shift-right: [w359] -> _
          shift-left: u8[][] [] -> [w358]
          shift-right: [w356] -> _
          shift-left: sgl[][] [] -> [w355]
          shift-right: [w353] -> _
          shift-left: u32 1 ("x") -> [w352]
          tunnel: [FALSE] -> w294
          stop <- w374 stop-if-true
          # "stop if (((finite samples == true) && (i == Nsamples)) || (stop == true))"
          n131 = Equal?(x=w379, y=w352) -> (x = y?=w378:bool)
          n132 = VISA Read(VISA resource name=w387, byte count=u32 1, error in (no error)=w388) -> (VISA resource name out=w384:refnum<visa-resource-name>, read buffer=w385:string, error out=w383:errorcluster)  [unwired: 1 out]
          n133 = And(x=w377, y=w378) -> (x .and. y?=w375:bool)
          n134 = case shown="\"#\"" w385 {
            tunnel: w384 -> [w414 w528 w540]
            tunnel: w383 -> [w413 w527 w539]
            tunnel: [w411 w525 w540] -> w382
            tunnel: [w410 w526 w539] -> w381
            tunnel: w380 -> [w407 w522 _]
            tunnel: [w415 w521 w538] -> w373
            tunnel: w372 -> [w415 w520 w538]
            tunnel: w371 -> [w406 w517 w536]
            tunnel: w370 -> [w401 w516 w537]
            tunnel: [w405 w517 w536] -> w369
            tunnel: [w400 w516 w537] -> w368
            tunnel: w367 -> [w412 _ _]
            tunnel: w366 -> [_ w515 _]
            tunnel: w365 -> [w404 _ _]
            tunnel: [w403 FALSE ("Clock drift") FALSE ("Clock drift")] -> w364
            tunnel: w354 -> [w402 _ _]
            tunnel: [w399 w513 w534] -> w363
            tunnel: w362 -> [w398 w513 w534]
            tunnel: w361 -> [w397 _ _]
            tunnel: [w396 w511 w532] -> w360
            tunnel: w357 -> [w395 w511 w532]
            tunnel: [w394 w512 w533] -> w359
            tunnel: w358 -> [w393 w512 w533]
            tunnel: [w392 w510 w531] -> w356
            tunnel: w355 -> [w391 w510 w531]
            tunnel: [w390 w509 w530] -> w353
            tunnel: w352 -> [w389 w509 w530]
            frame "#" {
              # "Mode case"
              n135 = VISA Read(VISA resource name=w414, byte count=w412, error in (no error)=w413) -> (VISA resource name out=w411:refnum<visa-resource-name>, read buffer=w409:string, error out=w410:errorcluster)  [unwired: 1 out]
              n136 = local read "Active pressure sensor constants"() -> (w408:T7[])
              n137 = case shown="0, Default" w402 {
                tunnel: w409 -> [w439 w482]
                tunnel: w408 -> [w438 w481]
                tunnel: w407 -> [w435 w478]
                tunnel: w406 -> [w434 w483]
                tunnel: [w433 w483] -> w405
                tunnel: w404 -> [w432 w477]
                tunnel: [w431 w476] -> w403
                tunnel: w401 -> [w440 w475]
                tunnel: [w440 w474] -> w400
                tunnel: [w430 w469] -> w399
                tunnel: w398 -> [w427 w465]
                tunnel: w397 -> [w429 w466]
                tunnel: [w425 w472] -> w396
                tunnel: w395 -> [w424 w470]
                tunnel: [w423 w473] -> w394
                tunnel: w393 -> [w422 w471]
                tunnel: [w421 w464] -> w392
                tunnel: w391 -> [w421 w463]
                frame 0, Default {
                  n138 = call "Process Data Buffer, Mode 0.vi"("DATA_Buffer excluding '#' [1...N]"=w439, "P constants"=w438) -> ("Pressures"=w419:sgl[], "Statuses"=w420:u8[], "dt_warn"=w436:u8)
                  n139 = Tick Count (ms)() -> (millisecond timer value=w418:u32)
                  n140 = Subtract(x=w418, y=w427) -> (x-y=w428:u32)
                  n141 = Greater Or Equal?(x=w428, y=w429) -> (x >= y?=w426:bool)
                  n142 = Bundle By Name(cluster=T8 {"Time Stamp"=timestamp(3537581686.1176577 s since 1904-01-01), "dt (us)"=0.0, "dt_warn"=0, "Pressures"=[], "Statuses"=[]} ("P data (Mode 0)"), "Time Stamp"=w435, "dt (us)"=w432, "dt_warn"=w436, "Pressures"=w419, "Statuses"=w420) -> (w416:T8)
                  n143 = Type Cast(type=FALSE ("Clock drift"), x=w436) -> (*(type *) &x=w431:bool)
                  n144 = case shown="True" w426 {
                    tunnel: [w447 w456] -> w430
                    tunnel: w427 -> [w447 _]
                    tunnel: w418 -> [_ w456]
                    tunnel: w419 -> [w446 w454]
                    tunnel: [w445 sgl[][] []] -> w425
                    tunnel: w424 -> [w444 w455]
                    tunnel: w420 -> [w443 w451]
                    tunnel: [w442 u8[][] []] -> w423
                    tunnel: w422 -> [w441 w452]
                    frame False {
                      n145 = Build Array (concatenate)(w441, w443) -> (w442:u8[][])
                      n146 = Build Array (concatenate)(w444, w446) -> (w445:sgl[][])
                    }
                    frame True {
                      n147 = Build Array (concatenate)(w452, w451) -> (→"Stale samples flag":u8[][])
                      n148 = Build Array (concatenate)(w455, w454) -> (→"Pressures time trace":sgl[][])
                    }
                  }
                  n149 = Build Array (concatenate)(w434, w416) -> (w433:T8[])
                }
                frame 1 {
                  n150 = call "Process Data Buffer, Mode 1.vi"("DATA_Buffer excluding '#' [1...N]"=w482, "P constants"=w481) -> ("Pressures (Pa)"=w460:sgl[], "Sensor temps (degC)"=w462:sgl[], "Statuses"=w461:u8[], "dt_warn"=w479:u8)
                  n151 = Tick Count (ms)() -> (millisecond timer value=w459:u32)
                  n152 = Subtract(x=w459, y=w465) -> (x-y=w468:u32)
                  n153 = Greater Or Equal?(x=w468, y=w466) -> (x >= y?=w467:bool)
                  n154 = Bundle By Name(cluster=T11 {"Time Stamp"=timestamp(3537581686.1176577 s since 1904-01-01), "dt (us)"=0.0, "dt_warn"=0, "Pressures"=[], "Die temps."=[], "Statuses"=[]} ("P data (Mode 1)"), "Time Stamp"=w478, "dt (us)"=w477, "dt_warn"=w479, "Pressures"=w460, "Statuses"=w461, "Die temps."=w462) -> (w457:T11)
                  n155 = Type Cast(type=FALSE ("Clock drift"), x=w479) -> (*(type *) &x=w476:bool)
                  n156 = case shown="True" w467 {
                    tunnel: [w493 w506] -> w469
                    tunnel: w465 -> [w493 _]
                    tunnel: w459 -> [_ w506]
                    tunnel: w460 -> [w492 w504]
                    tunnel: [w491 sgl[][] []] -> w472
                    tunnel: w470 -> [w490 w505]
                    tunnel: w461 -> [w489 w501]
                    tunnel: [w488 u8[][] []] -> w473
                    tunnel: w471 -> [w487 w502]
                    tunnel: [w486 sgl[][] []] -> w464
                    tunnel: w462 -> [w485 w497]
                    tunnel: w463 -> [w484 w498]
                    frame False {
                      n157 = Build Array (concatenate)(w487, w489) -> (w488:u8[][])
                      n158 = Build Array (concatenate)(w490, w492) -> (w491:sgl[][])
                      n159 = Build Array (concatenate)(w484, w485) -> (w486:sgl[][])
                    }
                    frame True {
                      n160 = Build Array (concatenate)(w502, w501) -> (w495:u8[][])
                      n161 = Build Array (concatenate)(w505, w504) -> (w494:sgl[][])
                      n162 = Build Array (concatenate)(w498, w497) -> (→"Sensor temperatures time trace (Mode \"P & T\" only)":sgl[][])
                      n163 = local write "Stale samples flag"(w495) -> ()
                      n164 = local write "Pressures time trace"(w494) -> ()
                    }
                  }
                  n165 = Build Array (concatenate)(w475, w457) -> (w474:T11[])
                }
              }
              n166 = Increment(x=w389) -> (x+1=w390:u32)
              "Samples acquired" <- w389
            }
            frame "$" {
              n167 = local read "AccelGyro constants"() -> (w523:T3)
              n168 = VISA Read(VISA resource name=w528, byte count=u32 29, error in (no error)=w527) -> (VISA resource name out=w525:refnum<visa-resource-name>, read buffer=w524:string, error out=w526:errorcluster)  [unwired: 1 out]
              n169 = call "Process State Buffer.vi"("AccelGyro constants"=w523, "STATE_Buffer excluding '$' [1...30]"=w524) -> ("Inertial state values"=w518:T4, "Environmental state values"=w519:T5)
              "Environmental state values" <- w519
              "Inertial state values" <- w518
              n170 = Bundle By Name(cluster=T9 {"Time Stamp"=timestamp(0 s since 1904-01-01), "dt (ms)"=0, "Environmental state values"={"Thermistor (degC)"=0.0, "Sensor temp. (degC)"=0.0, "P_atmos (Pa)"=0.0, "Rel. Humidity (%)"=0.0, "Density (kg/m^3)"=0.0, "Dew point (degC)"=0.0, "Pressure alt. (m)"=0.0, "Density alt. (m)"=0.0}, "Inertial state values"={"w_x (dps)"=0.0, "w_y (dps)"=0.0, "w_z (dps)"=0.0, "a_x (g)"=0.0, "a_y (g)"=0.0, "a_z (g)"=0.0, "Stale sample"=0, "Sensor temp. (degC)"=0.0}} ("All state values"), "Time Stamp"=w522, "dt (ms)"=w515, "Environmental state values"=w519, "Inertial state values"=w518) -> (w507:T9)
              n171 = Build Array (concatenate)(w520, w507) -> (w521:T9[])
            }
            frame Default {
            }
          }
          "Clock drift" <- w364
          n172 = Or(x="Stop streaming", y=w375) -> (x .or. y?=w374:bool)
        }
        n173 = Reciprocal(x=w334) -> (1/x=w309:dbl)
        n174 = property on="Pressures time trace" class="WFChart (strict)"("XScale.Multiplier"=w309) -> ()  [unwired: 2 in, 2 out]
        n175 = property on="Sensor temperatures time trace (Mode \"P & T\" only)" class="WFChart (strict)"("XScale.Multiplier"=w309) -> ()  [unwired: 2 in, 2 out]
        n176 = local write "Streaming"(w294) -> ()
        n177 = call "Stop data stream (s).vi"("VISA resource name in"=w329, "Error In"=w330) -> ("VISA resource name out"=w327:refnum<visa-resource-name>, "Error out"=w328:errorcluster)  [unwired: 7 in]
        n178 = call "Clear buffer.vi"("Error in"=w328, "dt for timeout (ms)"=w325, "VISA resource name in"=w327) -> ("Error out"=w297:errorcluster, "VISA resource name out"=w298:refnum<visa-resource-name>)  [unwired: 3 in]
        n179 = call "Close serial port.vi"("Error in"=w297, "VISA resource name"=w298) -> ("Error out"=w340:errorcluster)  [unwired: 9 in]
      }
      frame "T" {
        n180 = Divide(x=1000000.0, y=w549) -> (x/y=w542:dbl)
        n181 = call "Open serial port.vi"("VISA resource name"=w548) -> ("Error out"=w546:errorcluster, "VISA resource name out"=w547:refnum<visa-resource-name>)  [unwired: 9 in]
        n182 = call "Set stream dt (T).vi"("Error In"=w546, "dt (us)"=w542, "VISA resource name in"=w547) -> ("Error out"=w545:errorcluster, "ACK"=→"ACK 2":bool, "VISA resource name out"=w544:refnum<visa-resource-name>)  [unwired: 6 in]
        n183 = call "Close serial port.vi"("Error in"=w545, "VISA resource name"=w544) -> ("Error out"=w551:errorcluster)  [unwired: 9 in]
      }
      frame "t" {
        n184 = local read "Env. period (ms)"() -> (w556:i32)
        n185 = To Unsigned Long Integer(number=w556) -> (unsigned 32bit integer=w555:u32)
        n186 = call "Open serial port.vi"("VISA resource name"=w562) -> ("Error out"=w560:errorcluster, "VISA resource name out"=w561:refnum<visa-resource-name>)  [unwired: 9 in]
        n187 = call "Set state dt (t).vi"("Error In"=w560, "dt (ms)"=w555, "VISA resource name in"=w561) -> ("Error out"=w559:errorcluster, "ACK"=w557:bool, "VISA resource name out"=w558:refnum<visa-resource-name>)  [unwired: 6 in]
        n188 = call "Close serial port.vi"("Error in"=w559, "VISA resource name"=w558) -> ("Error out"=w564:errorcluster)  [unwired: 9 in]
        n189 = local write "ACK 2"(w557) -> ()
      }
      frame "M" {
        n190 = call "Open serial port.vi"("VISA resource name"=w568) -> ("Error out"=w574:errorcluster, "VISA resource name out"=w575:refnum<visa-resource-name>)  [unwired: 9 in]
        n191 = call "Set mode (M).vi"("Error In"=w574, "Mode"="Data mode", "VISA resource name in"=w575) -> ("Error out"=w573:errorcluster, "ACK"=w571:bool, "L_data"=→"L_data (bytes)":u16, "VISA resource name out"=w572:refnum<visa-resource-name>)  [unwired: 5 in]
        n192 = call "Close serial port.vi"("Error in"=w573, "VISA resource name"=w572) -> ("Error out"=w577:errorcluster)  [unwired: 9 in]
        n193 = local write "ACK 2"(w571) -> ()
      }
      frame "O" {
        n194 = call "Open serial port.vi"("VISA resource name"=w581) -> ("Error out"=w587:errorcluster, "VISA resource name out"=w588:refnum<visa-resource-name>)  [unwired: 9 in]
        n195 = call "Override maxSensorNum (O).vi"("Error In"=w587, "Max. number of sensors"="Max. num. sensors (override)", "VISA resource name in"=w588) -> ("Error out"=w586:errorcluster, "ACK"=→"ACK 3":bool, "L_data"=w582:u16, "VISA resource name out"=w585:refnum<visa-resource-name>)  [unwired: 5 in]
        n196 = local write "L_data (bytes)"(w582) -> ()
        n197 = call "Close serial port.vi"("Error in"=w586, "VISA resource name"=w585) -> ("Error out"=w590:errorcluster)  [unwired: 9 in]
      }
      frame "G" {
        n198 = call "Open serial port.vi"("VISA resource name"=w594) -> ("Error out"=w604:errorcluster, "VISA resource name out"=w605:refnum<visa-resource-name>)  [unwired: 9 in]
        n199 = call "Get status bits 1 (G).vi"("VISA resource name in"=w605, "Error In"=w604) -> ("nFaults"=w599:u8, "nSensors"=w598:u8, "nCards"=w597:u8, "PowerState"=w596:bool, "VISA resource name out"=w602:refnum<visa-resource-name>, "ACK"=→"ACK 5":bool, "Error out"=w603:errorcluster)  [unwired: 11 in]
        n200 = local read "System status"() -> (w595:T6)
        n201 = call "Close serial port.vi"("Error in"=w603, "VISA resource name"=w602) -> ("Error out"=w607:errorcluster)  [unwired: 9 in]
        n202 = Bundle By Name(cluster=w595, "Main power"=w596, "Occupied slots"=w597, "Active sensors"=w598, "Faulty sensors"=w599) -> (→"System status":T6)
      }
      frame "g" {
        w614 = T12."Disabled and Grayed Out" ("Disabled")
        w613 = T12."Enabled" ("Disabled")
        n203 = call "Open serial port.vi"("VISA resource name"=w611) -> ("Error out"=w626:errorcluster, "VISA resource name out"=w627:refnum<visa-resource-name>)  [unwired: 9 in]
        n204 = call "Get status bits 2 (g).vi"("VISA resource name in"=w627, "Error In"=w626) -> ("Mode"=w623:u8, "Therm_ok"=w615:bool, "BMI160_ok"=w619:bool, "BME280_ok"=w617:bool, "VISA resource name out"=w624:refnum<visa-resource-name>, "ACK"=w621:bool, "Error out"=w625:errorcluster)  [unwired: 11 in]
        n205 = Select(t=w613, s=w615, f=w614) -> (s? t:f=w618:T12)
        n206 = Select(t=w613, s=w617, f=w614) -> (s? t:f=w616:T12)
        n207 = stacked-sequence {
          tunnel: w618 -> [_ w634]
          tunnel: w616 -> [w633 _]
          tunnel: w615 -> [_ w635]
          frame #0 {
            n208 = property on="Environmental state values" class="Clust (strict)"("DisabledEnum"=w633) -> ()  [unwired: 2 in, 2 out]
            n209 = property on="Density (kg/m^3)" class="DigNum (strict)"("DisabledEnum"=w633) -> ()  [unwired: 2 in, 2 out]
            n210 = property on="Dew point (degC)" class="DigNum (strict)"("DisabledEnum"=w633) -> ()  [unwired: 2 in, 2 out]
            n211 = property on="Density alt. (m)" class="DigNum (strict)"("DisabledEnum"=w633) -> ()  [unwired: 2 in, 2 out]
          }
          frame #1 {
            n212 = case shown="False" w635 {
              tunnel: w634 -> [w636 _]
              frame False {
                n213 = property on="Density (kg/m^3)" class="DigNum (strict)"("DisabledEnum"=w636) -> ()  [unwired: 2 in, 2 out]
                n214 = property on="Dew point (degC)" class="DigNum (strict)"("DisabledEnum"=w636) -> ()  [unwired: 2 in, 2 out]
                n215 = property on="Density alt. (m)" class="DigNum (strict)"("DisabledEnum"=w636) -> ()  [unwired: 2 in, 2 out]
              }
              frame True {
              }
            }
            n216 = property on="Thermistor (degC)" class="DigNum (strict)"("DisabledEnum"=w634) -> ()  [unwired: 2 in, 2 out]
          }
        }
        n217 = local read "System status"() -> (w620:T6)
        n218 = call "Close serial port.vi"("Error in"=w625, "VISA resource name"=w624) -> ("Error out"=w629:errorcluster)  [unwired: 9 in]
        n219 = local write "ACK 5"(w621) -> ()
        n220 = Select(t=w613, s=w619, f=w614) -> (s? t:f=w612:T12)
        n221 = Bundle By Name(cluster=w620, "Env. sensor"=w617, "Inertial sensor"=w619, "Thermistor"=w615, "Mode"=w623) -> (w622:T6)
        n222 = property on="Inertial state values" class="Clust (strict)"("DisabledEnum"=w612) -> ()  [unwired: 2 in, 2 out]
        n223 = property on="AccelGyro constants" class="Clust (strict)"("DisabledEnum"=w612) -> ()  [unwired: 2 in, 2 out]
        n224 = property on="Accel. range (g)" class="Ring (strict)"("DisabledEnum"=w612) -> ()  [unwired: 2 in, 2 out]
        n225 = property on="Accel. rate (Hz)" class="Ring (strict)"("DisabledEnum"=w612) -> ()  [unwired: 2 in, 2 out]
        n226 = property on="Gyro. range (dps)" class="Ring (strict)"("DisabledEnum"=w612) -> ()  [unwired: 2 in, 2 out]
        n227 = property on="Gyro. rate (Hz)" class="Ring (strict)"("DisabledEnum"=w612) -> ()  [unwired: 2 in, 2 out]
        n228 = property on="ACK 8" class="Bool (strict)"("DisabledEnum"=w612) -> ()  [unwired: 2 in, 2 out]
        n229 = local write "System status"(w622) -> ()
      }
      frame "F" {
        n230 = call "Open serial port.vi"("VISA resource name"=w637) -> ("Error out"=w641:errorcluster, "VISA resource name out"=w642:refnum<visa-resource-name>)  [unwired: 9 in]
        n231 = call "Collate faulty sensor indices.vi"("Error In"=w641, "VISA resource name in"=w642) -> ("Error out"=w640:errorcluster, "Faulty sensor indices"=→"Faulty sensors":i32[], "VISA resource name out"=w639:refnum<visa-resource-name>)  [unwired: 7 in]
        n232 = call "Close serial port.vi"("Error in"=w640, "VISA resource name"=w639) -> ("Error out"=w644:errorcluster)  [unwired: 9 in]
      }
      frame "A" {
        n233 = call "Open serial port.vi"("VISA resource name"=w648) -> ("Error out"=w652:errorcluster, "VISA resource name out"=w653:refnum<visa-resource-name>)  [unwired: 9 in]
        n234 = call "Collate active sensor indices.vi"("Error In"=w652, "VISA resource name in"=w653) -> ("Error out"=w651:errorcluster, "Active sensor indices"=→"Active sensors":i32[], "VISA resource name out"=w650:refnum<visa-resource-name>)  [unwired: 7 in]
        n235 = call "Close serial port.vi"("Error in"=w651, "VISA resource name"=w650) -> ("Error out"=w655:errorcluster)  [unwired: 9 in]
      }
      frame "C" {
        n236 = call "Open serial port.vi"("VISA resource name"=w659) -> ("Error out"=w671:errorcluster, "VISA resource name out"=w672:refnum<visa-resource-name>)  [unwired: 9 in]
        n237 = call "Configure BMI160 (C).vi"("VISA resource name in"=w672, "Accel. range (g)"="Accel. range (g)", "Accel. rate (Hz)"="Accel. rate (Hz)", "Gyro. range (dps)"="Gyro. range (dps)", "Gyro. rate (Hz)"="Gyro. rate (Hz)", "Error In"=w671) -> ("VISA resource name out"=w669:refnum<visa-resource-name>, "ACK ok"=→"ACK 4":bool, "Error out"=w670:errorcluster)  [unwired: 11 in]
        n238 = case shown="0, Default" "Accel. range (g)" {
          tunnel: [sgl 2.0 ("accRange") sgl 4.0 ("accRange") sgl 8.0 ("accRange") sgl 16.0 ("accRange")] -> w663
          frame 0, Default {
          }
          frame 1 {
          }
          frame 2 {
          }
          frame 3 {
          }
        }
        n239 = case shown="0, Default" "Gyro. range (dps)" {
          tunnel: [sgl 125.0 ("accRange") sgl 250.0 ("accRange") sgl 500.0 ("accRange") sgl 1000.0 ("accRange") sgl 2000.0 ("accRange")] -> w661
          frame 0, Default {
          }
          frame 1 {
          }
          frame 2 {
          }
          frame 3 {
          }
          frame 4 {
          }
        }
        n240 = call "Close serial port.vi"("Error in"=w670, "VISA resource name"=w669) -> ("Error out"=w674:errorcluster)  [unwired: 9 in]
        n241 = local read "AccelGyro constants"() -> (w660:T3)
        n242 = Bundle By Name(cluster=w660, "accRange"=w663, "gyrRange"=w661) -> (w665:T3)
        n243 = local write "AccelGyro constants"(w665) -> ()
      }
      frame "Z" {
        n244 = call "Open serial port.vi"("VISA resource name"=w687) -> ("Error out"=w691:errorcluster, "VISA resource name out"=w692:refnum<visa-resource-name>)  [unwired: 9 in]
        n245 = call "Get Serial Number (Z).vi"("VISA resource name in"=w692, "Error In"=w691) -> ("VISA resource name out"=w689:refnum<visa-resource-name>, "Serial Number"=→"Serial no.":u16, "Error out"=w690:errorcluster)  [unwired: 5 in, 1 out]
        n246 = call "Close serial port.vi"("Error in"=w690, "VISA resource name"=w689) -> ("Error out"=w694:errorcluster)  [unwired: 9 in]
      }
      frame "D" {
        # "write after interval has passed, else append"
        n247 = local read "AccelGyro constants"() -> (w706:T3)
        n248 = call "Open serial port.vi"("VISA resource name"=w698) -> ("Error out"=w712:errorcluster, "VISA resource name out"=w713:refnum<visa-resource-name>)  [unwired: 9 in]
        n249 = call "Get Env data (oneshot) (D).vi"("VISA resource name in"=w713, "Error In"=w712) -> ("VISA resource name out"=w710:refnum<visa-resource-name>, "STATE_Buffer"=w709:string, "ACK"=→"ACK 6":bool, "Error out"=w711:errorcluster)  [unwired: 5 in]
        n250 = local read "Env. period (ms)"() -> (w701:i32)
        n251 = Get Date/Time In Seconds() -> (seconds since 1Jan1904=w699:timestamp)
        n252 = call "Close serial port.vi"("Error in"=w711, "VISA resource name"=w710) -> ("Error out"=w716:errorcluster)  [unwired: 9 in]
        n253 = String Subset(string=w709, offset (0)=1) -> (substring=w708:string)  [unwired: 1 in]
        n254 = call "Process State Buffer.vi"("AccelGyro constants"=w706, "STATE_Buffer excluding '$' [1...30]"=w708) -> ("Inertial state values"=w703:T4, "Environmental state values"=w704:T5)
        n255 = Bundle By Name(cluster=T9 {"Time Stamp"=timestamp(0 s since 1904-01-01), "dt (ms)"=0, "Environmental state values"={"Thermistor (degC)"=0.0, "Sensor temp. (degC)"=0.0, "P_atmos (Pa)"=0.0, "Rel. Humidity (%)"=0.0, "Density (kg/m^3)"=0.0, "Dew point (degC)"=0.0, "Pressure alt. (m)"=0.0, "Density alt. (m)"=0.0}, "Inertial state values"={"w_x (dps)"=0.0, "w_y (dps)"=0.0, "w_z (dps)"=0.0, "a_x (g)"=0.0, "a_y (g)"=0.0, "a_z (g)"=0.0, "Stale sample"=0, "Sensor temp. (degC)"=0.0}} ("All state values"), "Time Stamp"=w699, "dt (ms)"=w701, "Environmental state values"=w704, "Inertial state values"=w703) -> (w700:T9)
        n256 = local write "Environmental state values"(w704) -> ()
        n257 = local write "Inertial state values"(w703) -> ()
        n258 = Build Array (concatenate)(w714, w700) -> (w715:T9[])
      }
      frame "accgyr_consts" {
        n259 = call "Open serial port.vi"("VISA resource name"=w720) -> ("Error out"=w734:errorcluster, "VISA resource name out"=w735:refnum<visa-resource-name>)  [unwired: 9 in]
        n260 = call "Get AccelGyro constants (MCU EEPROM).vi"("VISA resource name in"=w735, "Error In"=w734) -> ("VISA resource name out"=w732:refnum<visa-resource-name>, "AccelGyro constants"=w729:T3, "ACK"=→"ACK 8":bool, "Error out"=w733:errorcluster)  [unwired: 5 in]
        n261 = Unbundle By Name(w729) -> ("gx offset"=w728:sgl, "gy offset"=w727:sgl, "gz offset"=w726:sgl, "ax offset"=w725:sgl, "ay offset"=w724:sgl, "az offset"=w723:sgl, "axyz scale"=w722:sgl)
        n262 = call "Close serial port.vi"("Error in"=w733, "VISA resource name"=w732) -> ("Error out"=w737:errorcluster)  [unwired: 9 in]
        n263 = Bundle By Name(cluster=T3 {"gyrRange"=125.0, "accRange"=2.0, "gx offset"=0.0, "gy offset"=0.0, "gz offset"=0.0, "ax offset"=0.0, "ay offset"=0.0, "az offset"=0.0, "axyz scale"=1.0} ("AccelGyro constants"), "gx offset"=w728, "gy offset"=w727, "gz offset"=w726, "ax offset"=w725, "ay offset"=w724, "az offset"=w723, "axyz scale"=w722) -> (→"AccelGyro constants":T3)
      }
      frame "EEPROM_Pconsts" {
        # "Must only run this case after running \"P\", \"G\", \"A\""
        n264 = local read "System status"() -> (w746:T6)
        n265 = Unbundle By Name(w746) -> ("Occupied slots"=w745:u8)
        n266 = To Long Integer(number=w745) -> (32bit integer=w744:i32)
        n267 = call "Open serial port.vi"("VISA resource name"=w741) -> ("Error out"=w751:errorcluster, "VISA resource name out"=w752:refnum<visa-resource-name>)  [unwired: 9 in]
        n268 = local read "Active sensors"() -> (w748:i32[])
        n269 = call "Concatenate all slot EEPROM arrays.vi"("Error In"=w751, "N slots occupied"=w744, "VISA resource name in"=w752) -> ("Error out"=w750:errorcluster, "ACK (all)"=→"ACK 7":bool, "All slot EEPROM values"=w743:T13[], "VISA resource name out"=w749:refnum<visa-resource-name>)  [unwired: 5 in]
        n270 = call "Populate pressure constants array.vi"("Occupied slot EEPROM values"=w743, "Active sensor indices"=w748) -> ("Active pressure sensor constants"=→"Active pressure sensor constants":T7[])
        n271 = call "Close serial port.vi"("Error in"=w750, "VISA resource name"=w749) -> ("Error out"=w754:errorcluster)  [unwired: 9 in]
      }
      frame "Exit", Default {
      }
    }
    n272 = Get Queue Status(queue=w241, return elements? (F)=FALSE, error in (no error)=w240) -> (queue out=w235:refnum<queue>, error out=w238:errorcluster, # elements in queue=w237:i32)  [unwired: 5 out]
    n273 = call <vilib>:"Clear Errors.vi"("error in (no error)"=w243, "specific error code to clear (0: all)"=1073676294) -> ("error out"=w242:errorcluster)  [unwired: 4 in, 1 out]
    "Error out" <- w242
    n274 = Equal To 0?(x=w237) -> (x = 0?=w236:bool)
  }
  "P data (mode 0)" <- w4
  n275 = Release Queue(queue=w10, error in (no error)=w16) -> (error out=w11:errorcluster)  [unwired: 1 in, 2 out]
  n276 = Merge Errors(w11, w12) -> (w13:errorcluster)
  n277 = local write "Error out"(w13) -> ()
